vi "Esclatometre_USB.vi"() -> ()   [LabVIEW 2017]
doc: "Esclatometre_USB - Versió Esclatòmetre feta sobre una base de Conus USB"
uses:
  Control 1.ctl
  Program Files/National Instruments/LabVIEW 2017/ProjectTemplates/Source/Core/Simple State Machine/controls/Data.ctl
  Program Files/National Instruments/LabVIEW 2017/ProjectTemplates/Source/Core/Simple State Machine/controls/StateEsclatometre.ctl
  <vilib>/DAQmx/read.llb/DAQmx Read (Digital 1D Bool NChan 1Samp 1Line).vi
  <vilib>/DAQmx/write.llb/DAQmx Write (Digital 1D Bool NChan 1Samp 1Line).vi
  <vilib>/DAQmx/miscellaneous.llb/DAQmx Fill In Error Info.vi
  Instance           2 17Saved   Conus_USB .vi
  Instance           1 17Saved   Conus_USB .vi
  Instance           4 17Saved   Conus_USB .vi
  <vilib>/Utility/file.llb/Write Delimited Spreadsheet (DBL).vi
panel:
  out "TextTemps":string
  out "TextDefor":string caption="TextDeformacio"
  out "FactorsUnitatsTermesInp_D":dbl[](array[numeric]) caption="FactorsUnitatsPendents_D"
  out "FactorsUnitatsTermesInd":dbl[](array[numeric]) caption="FactorsUnitatsPendents_F"
  out "TermesInd":dbl[](array[numeric]) caption="Pendents" format="%#_8g"
  in  "BtMaxD":bool caption="BtMaxF"
  out "MaximDaFmax":sgl caption="Maxim"
  out "ArraiMaxF_D":dbl[][](array[numeric])
  out "ArraiMaxims":sgl[](array[numeric])
  in  "Activa cilindre":bool
  out "data 2":bool[](array[boolean])
  out "Calibrar":bool
  out "Paro Emergencia":bool caption="Emergencia"
  out "Valor de control Paro Rotura":dbl caption="Valor de control sobrecarga"
  out "data":bool[](array[boolean])
  out "Data":T1
  out "Cilindre":bool caption="Pujar"
  in  "Rep. Fetes":u8 caption="N. Rep."
  in  "Salir":bool
  in  "EtiquetaTipusParo":string caption="N. Rep."
  in  "Etiqueta Velocitats":string caption="Presión"
  out "appended array":refnum<vi>[](array[refnum])
  out "MissatgesUsuari":string[](array[string])
  out "Caselles":refnum<vi>[](array[refnum])
  out "StringsEstatMáquina":string[](array[string])
  out "ParoDefor":bool caption="ParoRotura"
  out "ParoDeforFet":bool caption="ParoProcessat"
  out "ParoCargaFet":bool caption="ParoProcessat"
  out "ParoCarga":bool caption="ParoProcessat"
  in  "CaptadorD":u16(ring) caption="Unidades" items=["Tiempo"]
  in  "ActivaParoRotura":T2
  in  "ValorParoRotura":sgl caption="Rotura (%)" min=0 format="%#_3f"
  out "Ensayo activo":bool caption="Prueba en curso"
  out "ArraiMostresxProva":dbl[](array[numeric])
  out "NMostres":dbl
  in  "BtEliminarUltima":bool=TRUE caption="Eliminar última"
  out "Estado ensayo:":string caption="Tiempo"
  out "CodiAturada":u32
  out "ViuMotor":bool
  out "MotorBipolar":bool
  out "Baixar":bool
  out "Pujar":bool
  out "PrimerCaptador":i32
  out "rings":refnum<vi>[](array[refnum])
  in  "IndexUnitatsD":u8
  in  "IndexUnitatsF":u8
  in  "IndexCaptadorD":u8
  in  "IndexCaptadorF":u8
  out "EtiquetesRegistre":string[](array[string])
  out "Active_motor":bool
  in  "IniciAssaig":bool caption="Inici x Boto"
  out "DeforActiu":bool caption="Extensòmetre Pot."
  out "ValorSenseTara":dbl
  in  "VelocitatMàxima":dbl
  in  "BtMaxF":bool
  in  "CaptadorF":u16(ring) caption="Unidades" items=["P-40 bar"=22, "No presente"=25]
  in  "UnidadesF":u16(ring) caption="Unidades" items=["bar"=7, "kg/cm2"=8]
  in  "BtTaraF":bool caption="TARA"
  out "Fuerza":sgl caption="Presión" format="%.2f"
  out "Nº Tests":u8 caption="Tests:"
  out "Sobrecarga":bool
  out "Paro Manual":bool
  out "FCI":bool caption="FCR"
  out "FCS":bool caption="FCA"
  in  "ResoExten":i8(ring) caption="Resolució Extensometre" items=["0.1", "0.2", "0.5", "0.01", "0.02", "0.05", "0.001", "0.002", "0.005"]
  out "PrecargaOn":bool
  in  "ValorPrecarga":dbl caption="Precarga (%)"
  out "Calibratge D":dbl[](array[numeric])
  in  "UnidadesD":u16(ring) caption="Unidades" items=["sg"]
  in  "BtTaraD":bool caption="TARA"
  out "Deformacion":sgl caption="Tiempo" format="%.1f"
  out "Celula_0":u8
  in  "Células":u8(ring) caption="Célula 1" items=["0.5 kg", "1 Kg", "2 Kg", "5 kg", "10 kg", "20 kg", "50 kg", "100 kg", "200 kg", "300 kg", "500 kg", "1000 kg", "2000 kg", "5000 kg", "10000 kg", "20000 kg", "30000 kg", "P-20 kg", "P-200 kg", "P-500 kg", "P-5000 kg", "P-20000 kg", "P-40 bar", "P-60 bar", "P-20 bar", "No presente"]
  in  "UnidadesF_C2":u16(ring) caption="Unidades" items=["bar"=7]
  in  "UnidadesF_C1":u16(ring) caption="Unidades" items=["bar"=7, "kg/cm2"=8]
  out "ArraiUnitats":cluster{"String":string, "Value":u16}[](array[cluster])=[{"String"="kg", "Value"=0}, {"String"="N", "Value"=1}, {"String"="g", "Value"=2}, {"String"="daN", "Value"=3}, {"String"="cN", "Value"=4}, {"String"="KN", "Value"=5}, {"String"="lb", "Value"=6}]
  in  "UnitatsF":u8[](array[numeric])
  in  "Velocidad Retorno":sgl caption="Retorno" min=1 max=240 step=1 format="%#.1f"
  in  "Velocidad Ensayo":sgl caption="Ensayo" min=0 max=240 step=1
  out "ValorSobrecargaC2":dbl
  out "Valor de control sobrecarga":dbl
  out "Calibratge":dbl[](array[numeric])
  in  "ParaAssaig":bool
  out "ParoProcessat":bool
  out "Salidas_mando":T3={"HI_down"=TRUE, " LO_down"=TRUE, "HI_up"=TRUE, "*"=TRUE, " LO_up"=TRUE, " start"=TRUE, " Ensayo_down"=TRUE, " Ensayo_up"=TRUE}
  out "TempsLectura":u32=150
  out "Maxim":sgl
  in  "Inhibicio":bool
  in  "Ensayonuevo":bool caption="Ensayo Nuevo"
  in  "Guardar":bool caption="Informe"
  out "Iniciar / Finalizar":bool=TRUE caption="Finalizar prueba"
  out "TablaFinal":dbl[][](array[numeric])
  out "Tabla":dbl[][](array[numeric])
  in  "Columna":i32
  out "Paro Emergencia":bool
  out "ParoRotura":bool
  out "AssaigMM":bool
  out "DSenseTara":sgl caption="Fuerza - N"
  out "FactorsUnitatsPendents_D":dbl[](array[numeric])
  out "ConversioUnitatsD":dbl[](array[numeric])=[1.0, 9.8756, 1000.0, 0.98]
  in  "DadesAdquirides":dbl[](array[numeric]) format="%#_8g"
  out "FactorsUnitatsPendents_F":dbl[](array[numeric])
  in  "LedAssaig":bool caption="Ensayo Preparado"
  out "BaixarMM":bool
  out "PujarMM":bool
  in  "TaraD":sgl
  in  "ValMax":bool
  out "FSenseTara":sgl caption="Fuerza - N"
  in  "TaraF":sgl
  out "Password":string
  out "ValorSobrecargaC1":dbl
  out "ConversioUnitatsF":dbl[](array[numeric])=[1.0, 9.8756, 2.2]
  out "Pendents":dbl[](array[numeric]) format="%#_8g"
  in  "Procesa datos":bool
  in  "Stop":bool=TRUE
  in  "First time":bool
  out "?":cluster{"Y":dbl[], "Y":dbl[]}[](graph)
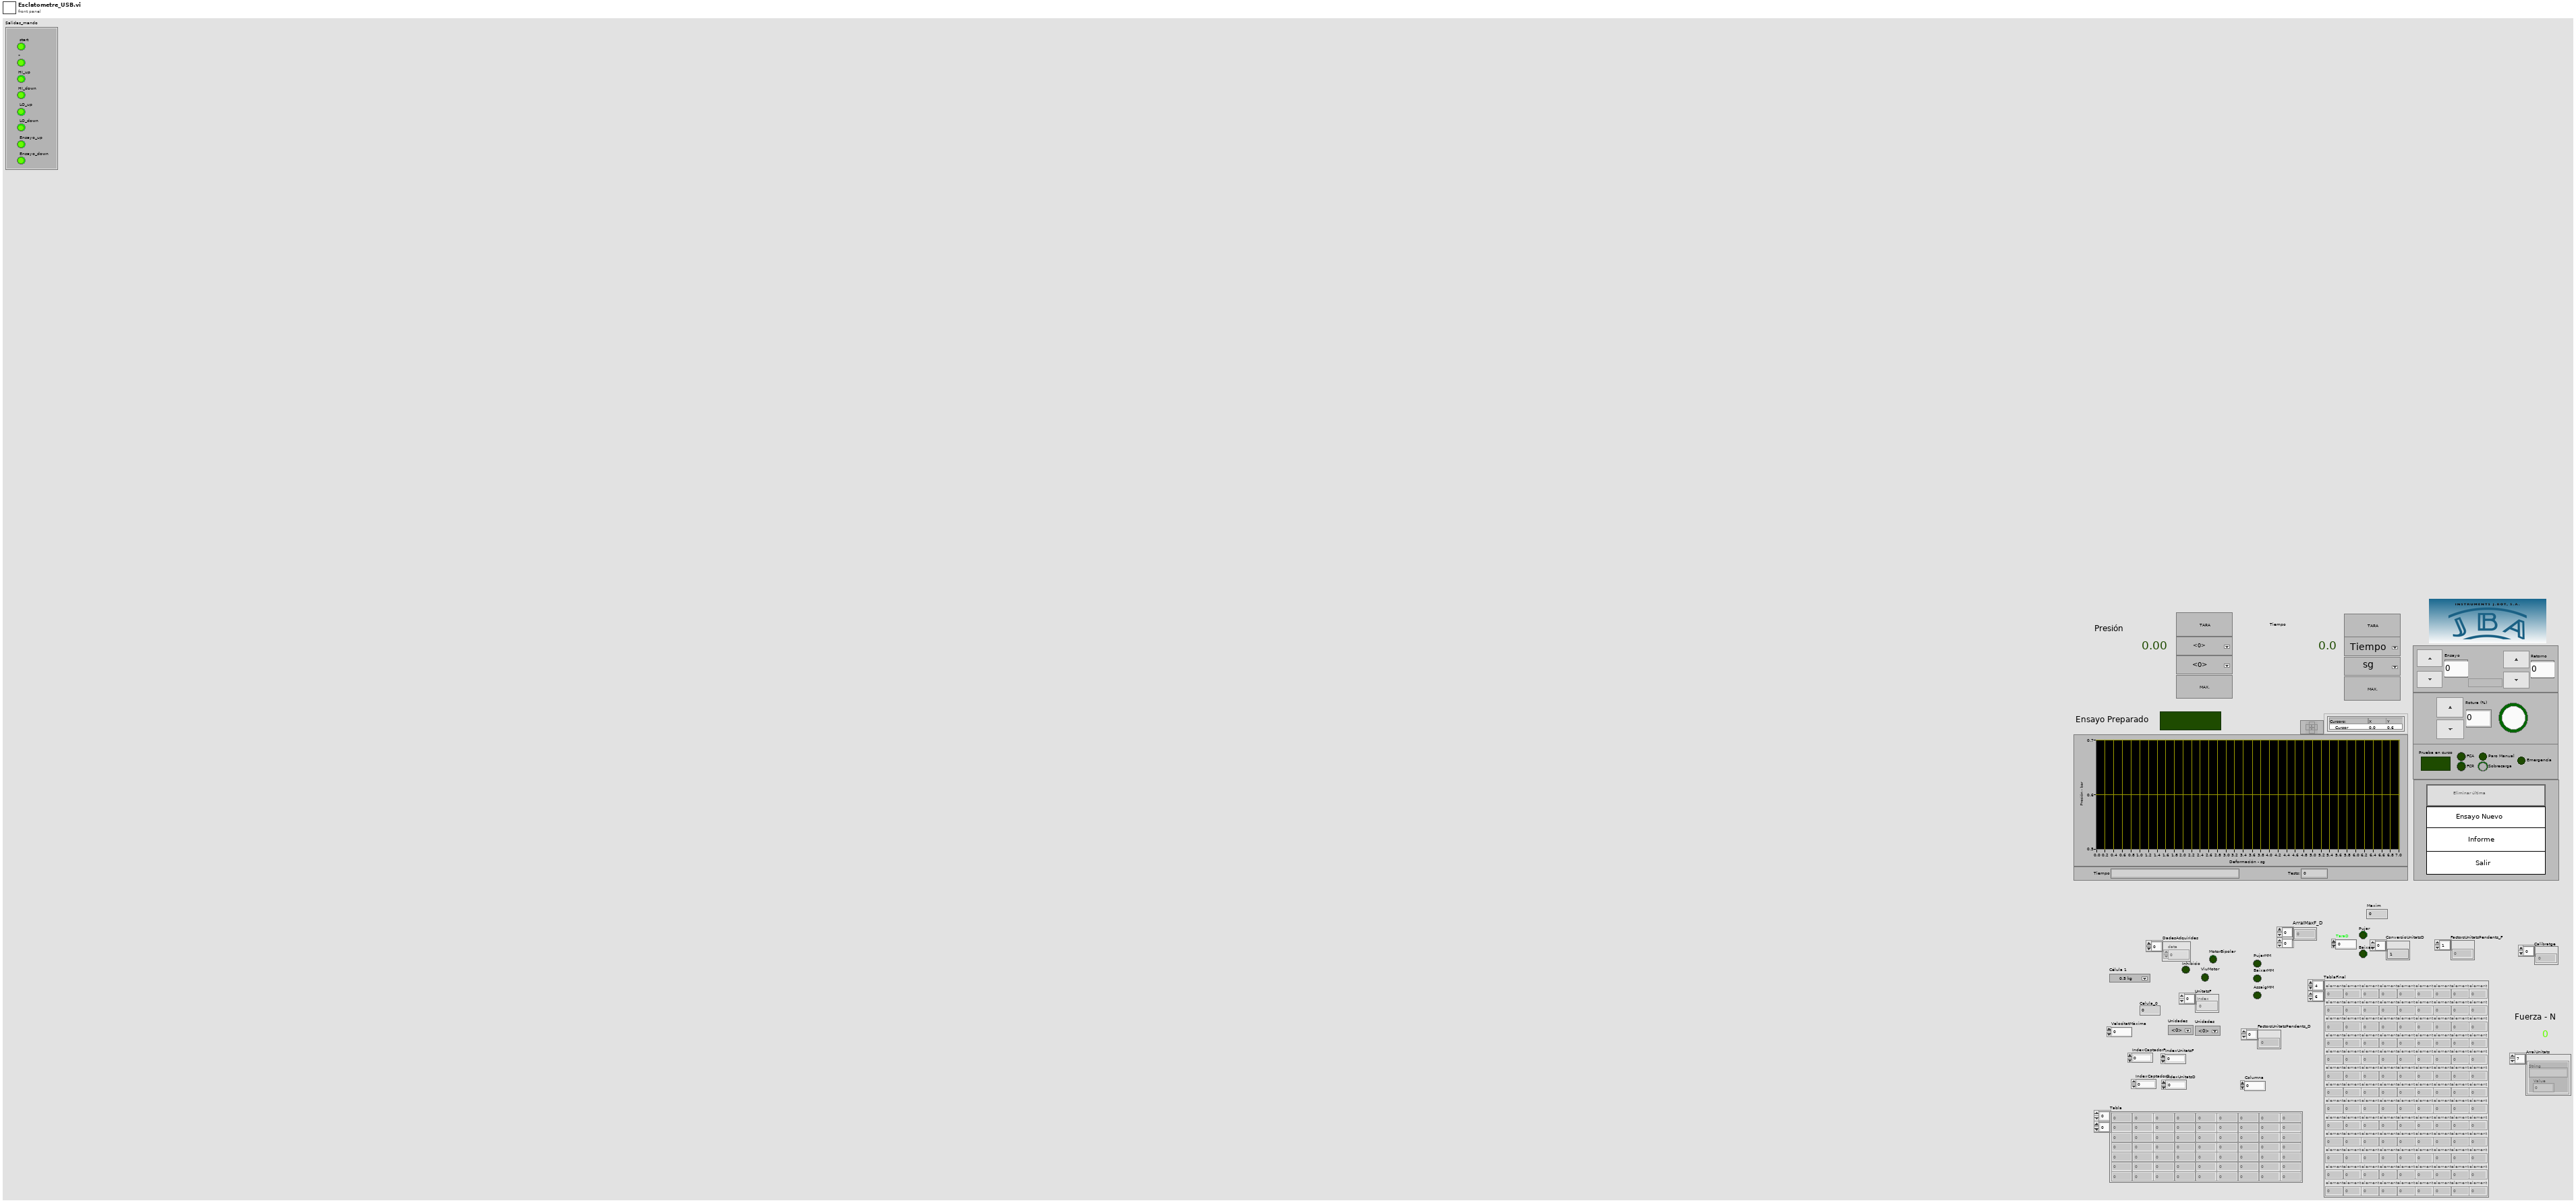
[diagram p1: front panel]
types:
  T1 = typedef "Data.ctl" = cluster{"Boolean <Replace Me>":bool, "String <Replace Me>":string, "Numeric <Replace Me>":dbl}
  T2 = typedef "Control 1.ctl" = bool
  T3 = cluster{"HI_down":bool, " LO_down":bool, "HI_up":bool, "*":bool, " LO_up":bool, " start":bool, " Ensayo_down":bool, " Ensayo_up":bool}
  T4 = typedef "StateEsclatometre.ctl" = enum16{"Initialize", "Wait for Event", "EsperaAssaig", "IniciaAssaig", "Assaig", "FiAssaig", "Emergencia", "Exit"}
  T5 = typedef "LVStringsAndValuesArrayTypeDef_U8.ctl" = cluster{"String":string, "Value":u8}[]
  T6 = typedef "LVStringsAndValuesArrayTypeDef_U16.ctl" = cluster{"String":string, "Value":u16}[]
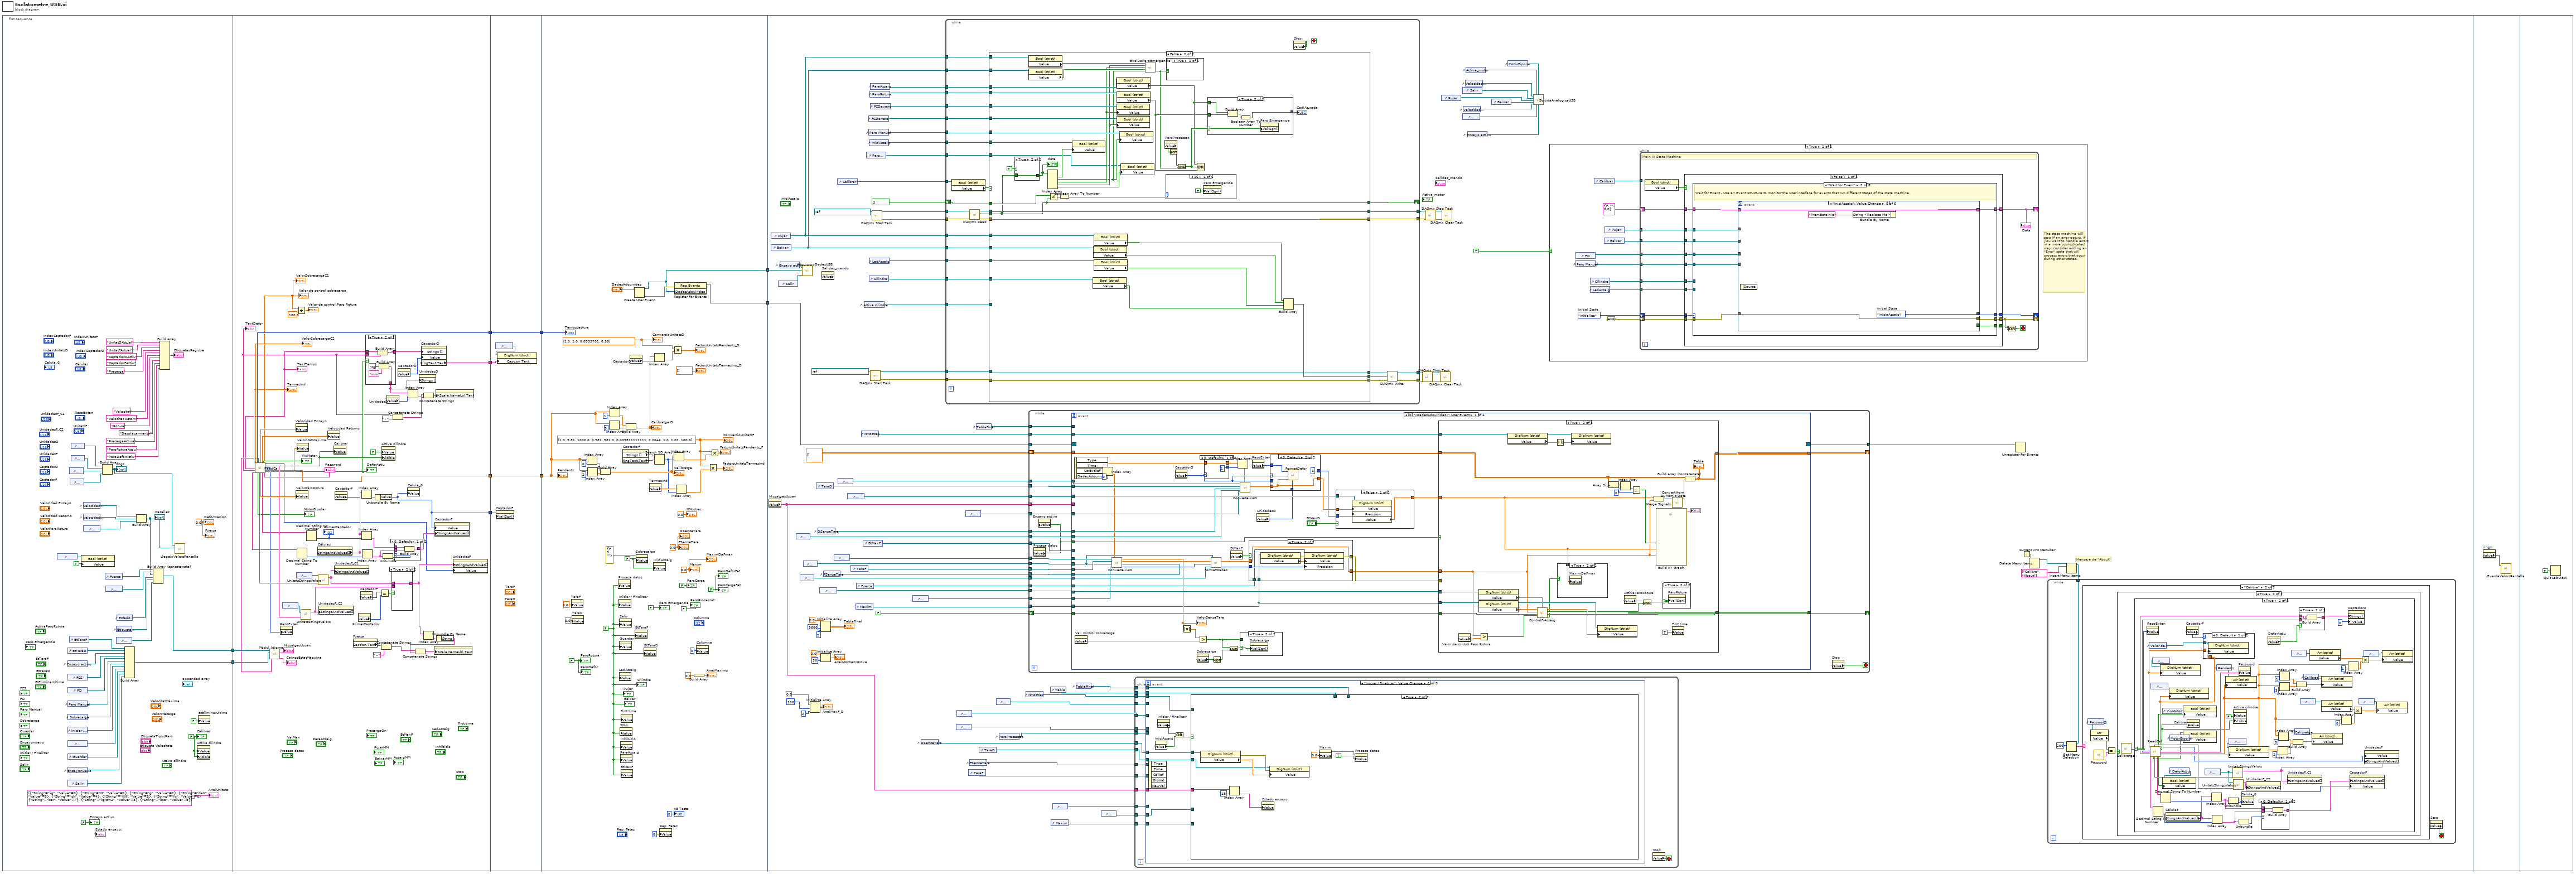
[diagram p0: block diagram]
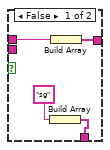
[diagram p3: hidden frame]
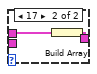
[diagram p4: hidden frame]
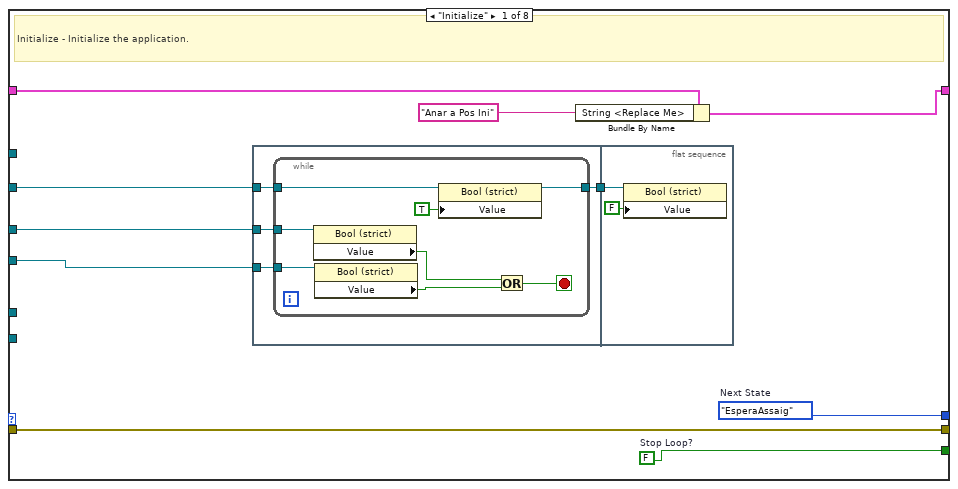
[diagram p6: hidden frame]
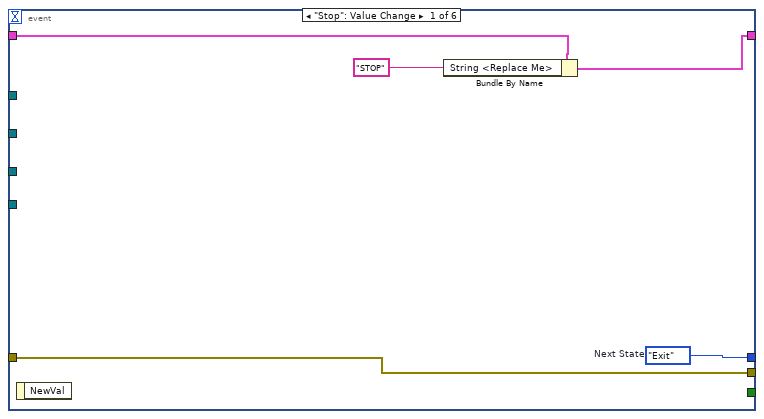
[diagram p7: hidden frame]
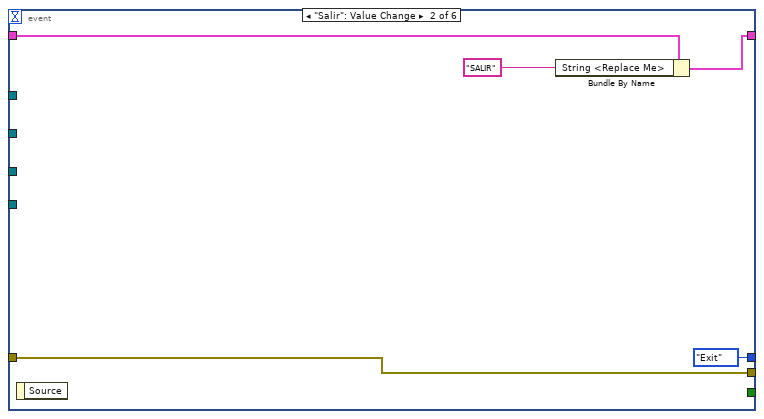
[diagram p8: hidden frame]
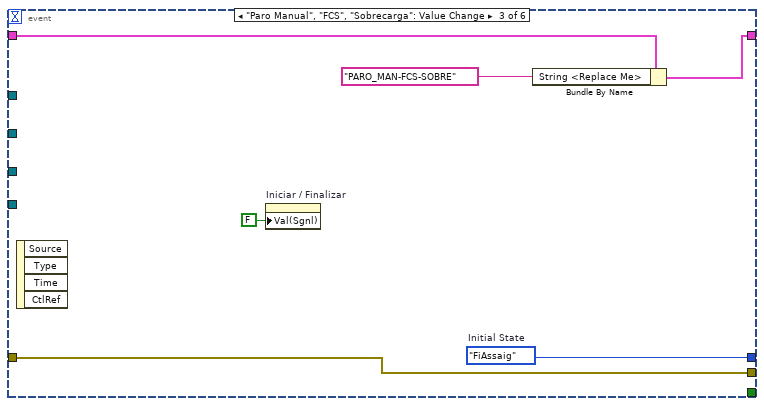
[diagram p9: hidden frame]
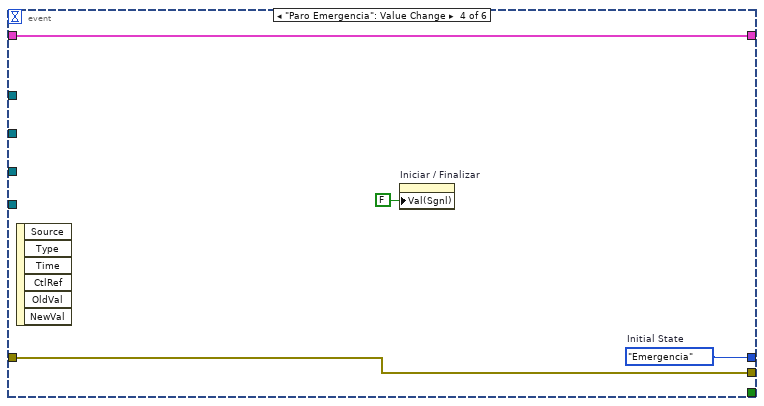
[diagram p10: hidden frame]
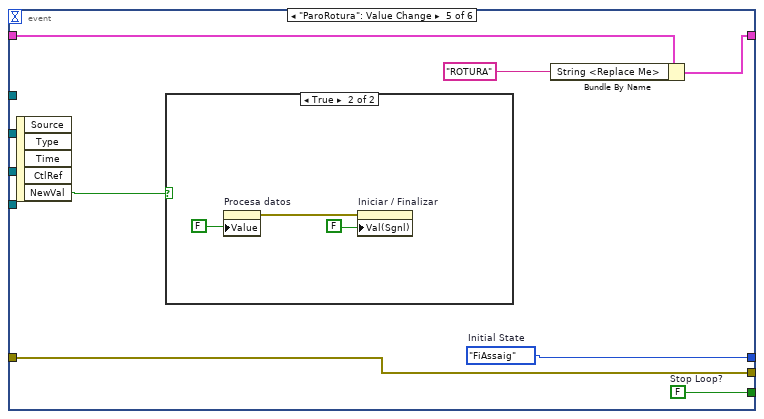
[diagram p11: hidden frame]
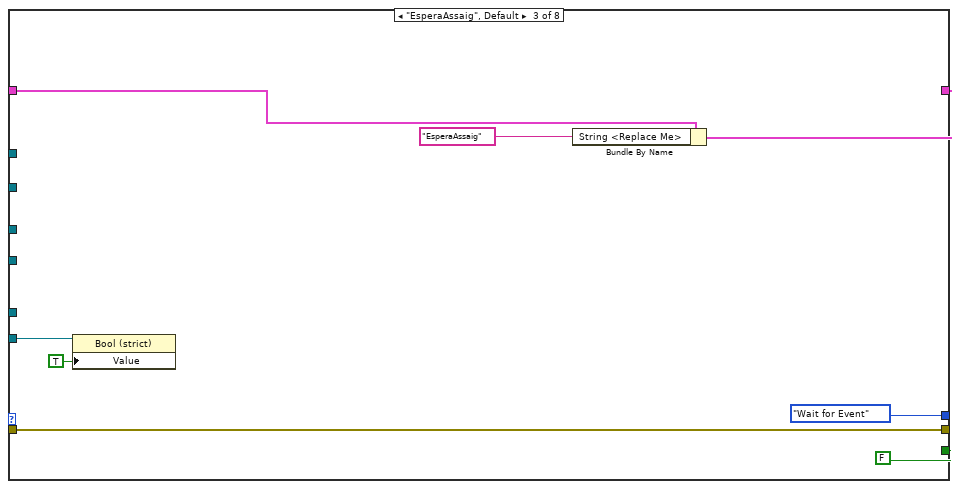
[diagram p13: hidden frame]
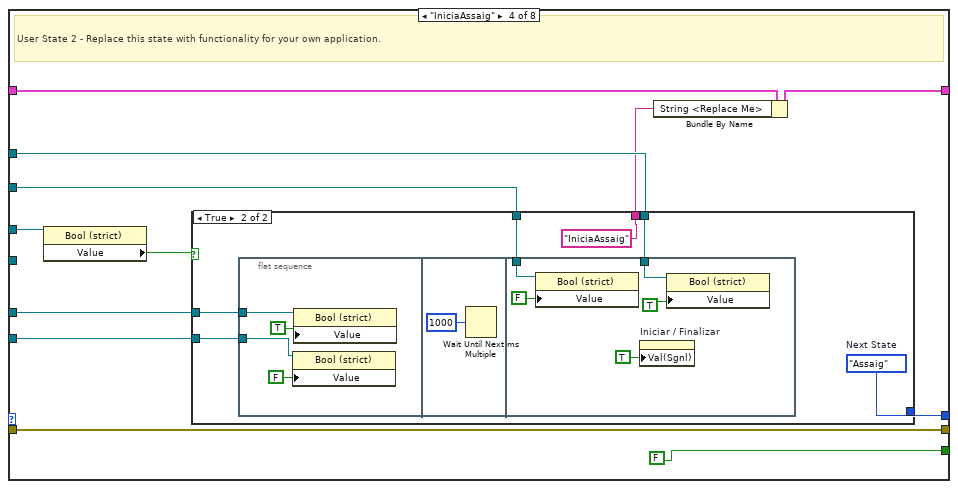
[diagram p14: hidden frame]
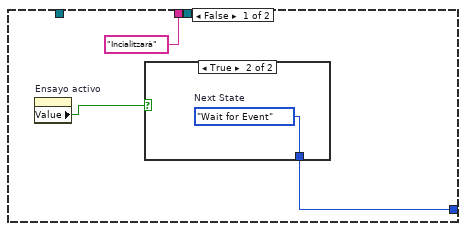
[diagram p15: hidden frame]
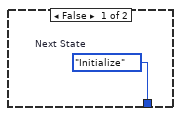
[diagram p16: hidden frame]
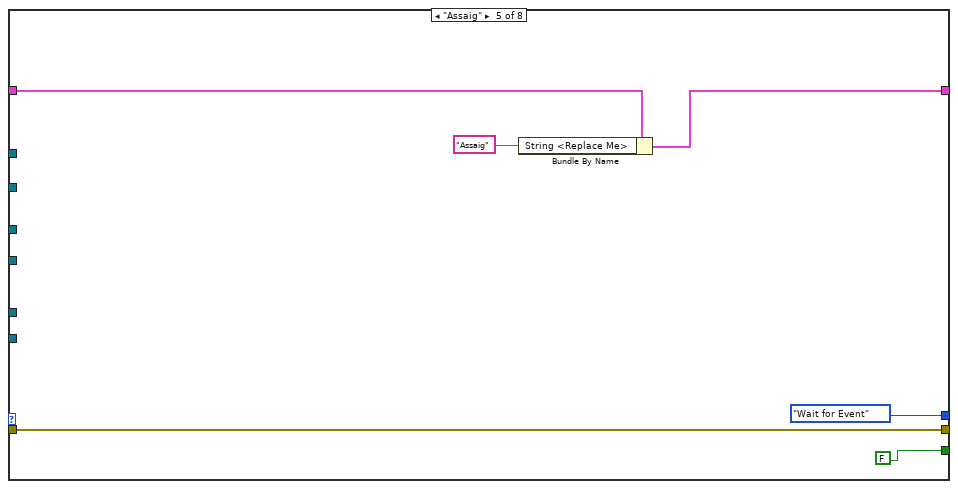
[diagram p17: hidden frame]
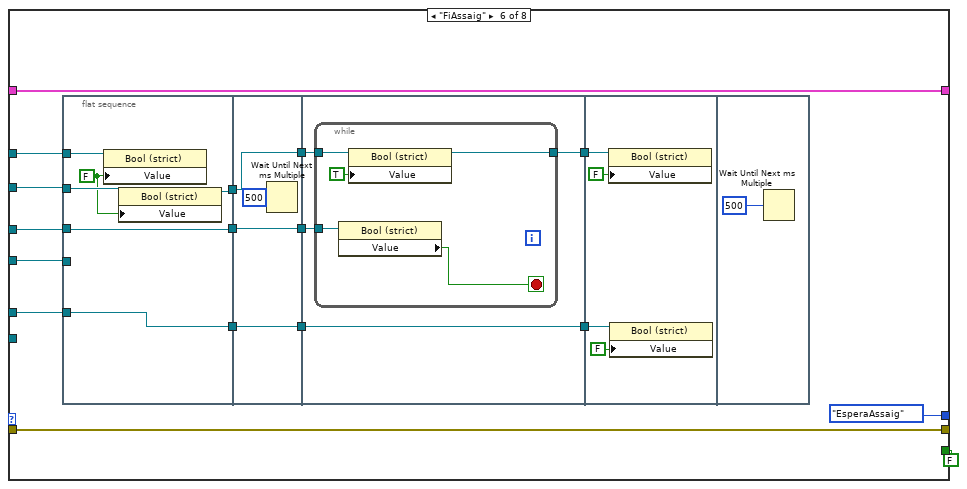
[diagram p18: hidden frame]
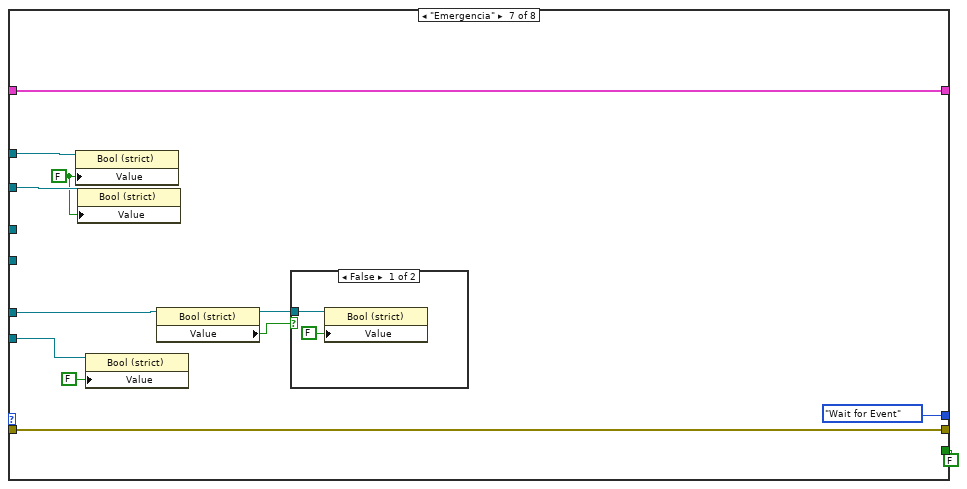
[diagram p19: hidden frame]
diagram:
  n1 = flat-sequence {
    tunnel: [w22] -> w3
    tunnel: [w21] -> w2
    tunnel: [w105] -> w10
    tunnel: [w118] -> w9
    tunnel: [w79] -> w4
    tunnel: w3 -> [w73]
    tunnel: w2 -> [w74]
    tunnel: [w58] -> w1
    tunnel: w10 -> [w142]
    tunnel: [w142] -> w8
    tunnel: w9 -> [w141]
    tunnel: [w141] -> w7
    tunnel: w4 -> [w140]
    tunnel: w1 -> [w138]
    tunnel: w8 -> [w167]
    tunnel: [w186] -> w6
    tunnel: [w178] -> w5
    tunnel: w7 -> [w177]
    tunnel: w6 -> [w276]
    tunnel: w5 -> [w258]
    frame #0 {
      w11 = FALSE ("Calibrar")
      w15 = sgl 0.0 ("Deformacion")
      (unwired) "CaptadorFActiu" ("value")
      n2 = control-ref of="ActivaParoRotura"() -> (w13:refnum<vi>)
      n3 = control-ref of="BtTaraD"() -> (w37:refnum<vi>)
      n4 = control-ref of="Ensayo activo"() -> (w36:refnum<vi>)
      n5 = control-ref of="FCS"() -> (w35:refnum<vi>)
      n6 = control-ref of="FCI"() -> (w34:refnum<vi>)
      n7 = control-ref of="Paro Manual"() -> (w33:refnum<vi>)
      n8 = control-ref of="Sobrecarga"() -> (w32:refnum<vi>)
      n9 = control-ref of="Iniciar / Finalizar"() -> (w31:refnum<vi>)
      n10 = control-ref of="BtEliminarUltima"() -> (w30:refnum<vi>)
      n11 = control-ref of="Guardar"() -> (w20:refnum<vi>)
      n12 = control-ref of="Ensayonuevo"() -> (w29:refnum<vi>)
      n13 = control-ref of="Salir"() -> (w28:refnum<vi>)
      n14 = control-ref of="BtTaraF"() -> (w38:refnum<vi>)
      n15 = control-ref of="CaptadorD"() -> (w42:refnum<vi>)
      n16 = control-ref of="CaptadorF"() -> (w41:refnum<vi>)
      n17 = control-ref of="UnidadesD"() -> (w44:refnum<vi>)
      n18 = control-ref of="UnidadesF"() -> (w43:refnum<vi>)
      n19 = property class="Bool (strict)"(reference=w13, "Value"=T2 TRUE) -> ()  [unwired: 1 in, 2 out]
      n20 = control-ref of="Velocidad Ensayo"() -> (w27:refnum<vi>)
      n21 = control-ref of="Velocidad Retorno"() -> (w45:refnum<vi>)
      n22 = control-ref of="ValorParoRotura"() -> (w26:refnum<vi>)
      n23 = Build Array(w44, w43, w42, w41) -> (w40:refnum<vi>[])
      "rings" <- w40
      n24 = control-ref of="Fuerza"() -> (w25:refnum<vi>)
      n25 = control-ref of="Deformacion"() -> (w24:refnum<vi>)
      n26 = control-ref of="Etiqueta Velocitats"() -> (w17:refnum<vi>)
      n27 = control-ref of="EtiquetaTipusParo"() -> (w16:refnum<vi>)
      n28 = control-ref of="Estado ensayo:"() -> (w18:refnum<vi>)
      n29 = Build Array(w38, w37, w36, w35, w34, w33, w32, w31, w30, w20, w29, w28) -> (w22:refnum<vi>[])
      n30 = Build Array(w27, w45, w26) -> (w19:refnum<vi>[])
      "Caselles" <- w19
      n31 = Build Array (concatenate)(w25, w24, w19, w18, w17, w16) -> (w21:refnum<vi>[])
      n32 = Build Array("UnitatDActual" ("value"), "UnitatFActual" ("value"), "CaptadorDActiu" ("value"), "Precarga" ("value"), "Velocitat" ("value"), "Velocitat Retorn" ("value"), "Rotura" ("value"), "Desplazamiento" ("value"), "PrecargaActiva" ("value"), "ParoRoturaActiu" ("value"), "ParoDeforActiu" ("value")) -> (→"EtiquetesRegistre":string[])
      n33 = call "LlegeixValorsPantalla.vi"("rings"=w40, "Caselles 2"=w19) -> ()  [unwired: 9 in]
      n34 = property on="Activa cilindre" class="Bool (strict)"("Value"=w11, "Visible"=w11) -> ()  [unwired: 2 in, 2 out]
      n35 = property on="BtEliminarUltima" class="Bool (strict)"("Value"=FALSE ("BtEliminarUltima")) -> ()  [unwired: 2 in, 2 out]
      "Ensayo activo" <- FALSE ("Ensayo activo")
      "Fuerza" <- w15
      "Deformacion" <- w15
      "ArraiUnitats" <- cluster{"String":string, "Value":u16}[] [{"String"="kg", "Value"=0}, {"String"="N", "Value"=1}, {"String"="g", "Value"=2}, {"String"="daN", "Value"=3}, {"String"="cN", "Value"=4}, {"String"="KN", "Value"=5}, {"String"="lb", "Value"=6}, {"String"="bar", "Value"=7}, {"String"="kg/cm2", "Value"=8}, {"String"="kpa", "Value"=9}] ("Strings And Values [] 2")
      "Calibrar" <- w11
    }
    frame #1 {
      n36 = call "ReadCal.vi"() -> ("SobrecargaC2"=→"ValorSobrecargaC2":dbl, "TermesInd"=→"TermesInd":dbl[], "ResoExten"=w104:i8, "TextTemps"=w60:string, "TextDefor"=w59:string, "SegonCaptador"=w111:string, "TempsLectura"=w118:u16, "Idioma"=w62:string, "MotorBipolar"=→"MotorBipolar":bool, "UnitatsC2"=w112:string, "UnitatsC1"=w113:string, "Velocitat"=w119:dbl, "ParoRotura"=w120:dbl, "V. Retorn"=w70:dbl, "PrimerCaptador"=w109:string, "ViuMotor"=→"ViuMotor":bool, "DeforActiva"=w63:bool, "Unidades"=w71:u8, "Calibrar"=w66:bool, "SobrecargaC1"=w69:dbl, "Password"=→"Password":string, "Pendents"=w105:dbl[], "VelocitatMàxima"=w102:dbl)  [unwired: 2 in, 3 out]
      "ValorSobrecargaC1" <- w69
      "Valor de control sobrecarga" <- w69
      "DeforActiu" <- w63
      "TextDefor" <- w59
      "TextTemps" <- w60
      n37 = call "Módul_Idioma.vi"("Idioma"=w62, "Array"=w73, "Caselles"=w74) -> ("TextosEstatMaquina"=→"StringsEstatMáquina":string[], "MissatgesUsuari"=→"MissatgesUsuari":string[])  [unwired: 7 in]
      n38 = property on="ResoExten" class="Ring (strict)"("Value"=w104) -> ()  [unwired: 2 in, 2 out]
      n39 = control-ref of="ArraiUnitats"() -> (w114:refnum<vi>)
      n40 = property on="Velocidad Ensayo" class="DigNum (strict)"("Value"=w119) -> ()  [unwired: 2 in, 2 out]
      n41 = property on="ValorParoRotura" class="DigNum (strict)"("Value"=w120) -> ()  [unwired: 2 in, 2 out]
      n42 = Divide(x=w69, y=100.0) -> (x/y=→"Valor de control Paro Rotura":dbl)
      n43 = control-ref of="ArraiUnitats"() -> (w115:refnum<vi>)
      n44 = property on="VelocitatMàxima" class="DigNum (strict)"("Value"=w102) -> ()  [unwired: 2 in, 2 out]
      n45 = Decimal String To Number(string=w111) -> (number=w110:i32)  [unwired: 2 in, 1 out]
      n46 = call "UnitatsStringsValors.vi"("UnitatsC1"=w112, "Arr Refnum"=w114) -> ("Array 2"=w88:cluster{"String":string, "Value":u16}[])  [unwired: 1 out]
      n47 = Decimal String To Number(string=w109) -> (number=w108:i32)  [unwired: 2 in, 1 out]
      "PrimerCaptador" <- w108
      n48 = property on="Células" class="Ring (strict)"() -> ("StringsAndValues[]"=w95:T5)  [unwired: 2 in, 2 out]
      n49 = call "UnitatsStringsValors.vi"("UnitatsC1"=w113, "Arr Refnum"=w115) -> ("Array 2"=w89:cluster{"String":string, "Value":u16}[])  [unwired: 1 out]
      n50 = property on="UnidadesF_C2" class="Ring (strict)"("StringsAndValues[]"=w88) -> ()  [unwired: 2 in, 2 out]
      n51 = property on="Velocidad Retorno" class="DigNum (strict)"("Value"=w70) -> ()  [unwired: 2 in, 2 out]
      n52 = property on="Calibrar" class="Bool (strict)"("Value"=w66) -> ()  [unwired: 2 in, 2 out]
      n53 = property on="UnidadesF_C1" class="Ring (strict)"("StringsAndValues[]"=w89) -> ()  [unwired: 2 in, 2 out]
      n54 = property on="CaptadorF" class="Ring (strict)"() -> ("Value"=w93:u16)  [unwired: 2 in, 2 out]
      n55 = property on="Fuerza" class="DigNum (strict)"() -> ("Caption.Text"=w100:string)  [unwired: 2 in, 2 out]
      n56 = property on="PrimerCaptador" class="DigNum (strict)"() -> ("Value"=w90:i32)  [unwired: 2 in, 2 out]
      n57 = property on="CaptadorF" class="Ring (strict)"() -> ("Value"=w91:u16)  [unwired: 2 in, 2 out]
      n58 = Index Array(array=w95, index=w93) -> (element=w94:cluster{"String":string, "Value":u8})
      n59 = Index Array(array=w95, index=w108) -> (element=w97:cluster{"String":string, "Value":u8})
      n60 = Index Array(array=w95, index=w110) -> (element=w106:cluster{"String":string, "Value":u8})
      n61 = case shown="True" w63 {
        tunnel: w60 -> [w123 w128]
        tunnel: [w126 w132] -> w84
        tunnel: w59 -> [_ w127]
        tunnel: [w124 w129] -> w61
        frame False {
          n62 = Build Array("sg") -> (w124:string[])
          n63 = Build Array(w123) -> (w126:string[])
        }
        frame True {
          n64 = Build Array(w128, w127) -> (w132:string[])
          n65 = Build Array("sg", "mm") -> (w129:string[])
        }
      }
      n66 = Unbundle By Name(w94) -> ("Value"=w79:u8)
      n67 = Equal?(x=w91, y=w90) -> (x = y?=w92:bool)
      n68 = Concatenate Strings(w100, " - ") -> (w99:string)
      n69 = property on="Activa cilindre" class="Bool (strict)"("Value"=FALSE ("ActivaCilindre"), "Visible"=w66) -> ()  [unwired: 2 in, 2 out]
      n70 = Unbundle(w106) -> ("Value"=w107:u8)  [unwired: 1 out]
      n71 = property on="UnidadesD" class="Ring (strict)"() -> ("Value"=w83:u16)  [unwired: 2 in, 2 out]
      n72 = case shown="True" w92 {
        tunnel: w89 -> [_ w122]
        tunnel: [w121 w122] -> w72
        tunnel: w88 -> [w121 _]
        frame False {
        }
        frame True {
        }
      }
      n73 = Concatenate Strings(w59, " - ") -> (w80:string)
      n74 = case shown="0, Default" w107 {
        tunnel: w97 -> [w135 w136]
        tunnel: w106 -> [w134 _]
        tunnel: [w133 w137] -> w96
        frame 0, Default {
          n75 = Build Array(w135, w134) -> (w133:cluster{"String":string, "Value":u8}[])
        }
        frame 17 {
          n76 = Build Array(w136) -> (w137:cluster{"String":string, "Value":u8}[])
        }
      }
      n77 = property on="CaptadorD" class="Ring (strict)"() -> ("Value"=w85:u16)  [unwired: 2 in, 2 out]
      n78 = property on="Celula_0" class="DigNum (strict)"("Value"=w79) -> ()  [unwired: 2 in, 2 out]
      n79 = Index Array(array=w61, index=w83) -> (element=w82:string)
      n80 = property on="UnidadesD" class="Ring (strict)"("Strings []"=w61) -> ()  [unwired: 2 in, 2 out]
      n81 = property on="CaptadorD" class="Ring (strict)"("Strings []"=w84, "Value"=w85) -> ("RingText.Text"=w58:string)  [unwired: 2 in, 2 out]
      n82 = Concatenate Strings(w80, w82) -> (w98:string)
      n83 = Index Array(array=w72) -> (element=w86:cluster{"String":string, "Value":u16})  [unwired: 1 in]
      n84 = property on="CaptadorF" class="Ring (strict)"("Value"=w79, "StringsAndValues[]"=w96) -> ()  [unwired: 2 in, 2 out]
      n85 = property class="XYGraph (strict)"("XScale.NameLbl.Text"=w98) -> ()  [unwired: 2 in, 2 out]
      n86 = Unbundle By Name(w86) -> ("String"=w87:string)
      n87 = Concatenate Strings(w99, w87) -> (w103:string)
      n88 = property class="XYGraph (strict)"("YScale.NameLbl.Text"=w103) -> ()  [unwired: 2 in, 2 out]
      n89 = property on="UnidadesF" class="Ring (strict)"("StringsAndValues[]"=w72, "Value"=w71) -> ()  [unwired: 2 in, 2 out]
    }
    frame #2 {
      n90 = control-ref of="Deformacion"() -> (w139:refnum<vi>)
      n91 = property on="CaptadorF" class="Ring (strict)"("Val(Sgnl)"=w140) -> ()  [unwired: 2 in, 2 out]
      n92 = property class="DigNum (strict)"(reference=w139, "Caption.Text"=w138) -> ()  [unwired: 1 in, 2 out]
    }
    frame #3 {
      w155 = FALSE ("ParoCargaFet")
      w149 = sgl 0.0 ("Maxim")
      w154 = FALSE ("ParoRotura")
      w165 = dbl[] [1.0, 1.0, 0.0393701, 0.98]
      w180 = sgl 0.0 ("FSenseTara")
      w148 = dbl[] [1.0, 9.81, 1000.0, 0.981, 981.0, 0.009811111111, 2.2046, 1.0, 1.02, 100.0]
      w160 = FALSE ("Sobrecarga")
      w152 = FALSE ("Iniciar / Finalizar")
      n93 = property on="TaraF" class="DigNum (strict)"("Value"=sgl 0.0 ("Tara")) -> ()  [unwired: 2 in, 2 out]
      n94 = property on="TaraD" class="DigNum (strict)"("Value"=sgl 0.0 ("TaraD")) -> ()  [unwired: 2 in, 2 out]
      n95 = Index Array(array=w167, index=0) -> (element=w173:dbl)
      n96 = Index Array(array=w167, index=2) -> (element=w174:dbl)
      n97 = Build Array(w173, w174) -> (w172:dbl[])
      "Calibratge" <- w172
      n98 = Index Array(array=w167, index=3) -> (element=w168:dbl)
      n99 = Index Array(array=w167, index=1) -> (element=w166:dbl)
      n100 = property on="Procesa datos" class="Bool (strict)"("Value"=w152) -> ()  [unwired: 2 in, 2 out]
      n101 = property on="Iniciar / Finalizar" class="Bool (strict)"("Value"=w152) -> ()  [unwired: 2 in, 2 out]
      n102 = property on="LedAssaig" class="Bool (strict)"("Value"=w152) -> ()  [unwired: 2 in, 2 out]
      n103 = property on="Salir" class="Bool (strict)"("Value"=w152) -> ()  [unwired: 2 in, 2 out]
      n104 = property on="Guardar" class="Bool (strict)"("Value"=w152) -> ()  [unwired: 2 in, 2 out]
      n105 = property on="Stop" class="Bool (strict)"("Value"=w152) -> ()  [unwired: 2 in, 2 out]
      n106 = property on="Inhibicio" class="Bool (strict)"("Value"=w152) -> ()  [unwired: 2 in, 2 out]
      n107 = property on="ParaAssaig" class="Bool (strict)"("Value"=w152) -> ()  [unwired: 2 in, 2 out]
      n108 = property on="First time" class="Bool (strict)"("Value"=w152) -> ()  [unwired: 2 in, 2 out]
      n109 = property on="BtMaxF" class="Bool (strict)"("Value"=w152) -> ()  [unwired: 2 in, 2 out]
      n110 = property on="CaptadorF" class="Ring (strict)"() -> ("Strings []"=w159:string[], "RingText.Text"=w158:string)  [unwired: 2 in, 2 out]
      n111 = Build Array(w166, w168) -> (w163:dbl[])
      "Calibratge D" <- w163
      n112 = property on="CaptadorD" class="Ring (strict)"() -> ("Value"=w164:u16)  [unwired: 2 in, 2 out]
      n113 = Create User Event(user event datatype="DadesAdquirides") -> (user event=w178:refnum<user-event>, error out=w185:errorcluster)  [unwired: 1 in]
      n114 = property on="BtTaraF" class="Bool (strict)"("Value"=w152) -> ()  [unwired: 2 in, 2 out]
      n115 = property on="Sobrecarga" class="Bool (strict)"(error in=errorcluster {"status"=FALSE, "code"=0, "source"=""} ("error in (no error)"), "Value"=w160) -> ()  [unwired: 1 in, 2 out]
      n116 = property on="BtTaraD" class="Bool (strict)"("Value"=w152) -> ()  [unwired: 2 in, 2 out]
      n117 = property on="TermesInd" class="Arr (strict)"() -> ("Value"=w146:dbl[])  [unwired: 2 in, 2 out]
      n118 = property on="IniciAssaig" class="Bool (strict)"("Value"=w160) -> ()  [unwired: 2 in, 2 out]
      n119 = Index Array(array=w163, index=w164) -> (element=w162:dbl)
      n120 = Search 1D Array(1D array=w159, element=w158) -> (index of element=w145:i32)  [unwired: 1 in]
      n121 = property on="Rep. Fetes" class="DigNum (strict)"("Value"=u8 0 ("Rep. Fetes")) -> ()  [unwired: 2 in, 2 out]
      n122 = Multiply(x=w165, y=w162) -> (x*y=→"FactorsUnitatsPendents_D":dbl[])
      n123 = Index Array(array=w172, index=w145) -> (element=w171:dbl)
      n124 = register-events(error in=w185, w178) -> (reference out=w186:refnum<event-registration>)  [unwired: 1 in, 1 out]
      n125 = Index Array(array=w146, index=w145) -> (element=w144:dbl)
      n126 = Build Array(0.0 ("element")) -> (→"ArraiMaxims":dbl[])
      n127 = property on="Columna" class="DigNum (strict)"("Value"=0 ("Columna")) -> ()  [unwired: 2 in, 2 out]
      n128 = Multiply(x=w148, y=w144) -> (x*y=→"FactorsUnitatsTermesInd":dbl[])
      n129 = Multiply(x=w148, y=w171) -> (x*y=→"FactorsUnitatsPendents_F":dbl[])
      "Pendents" <- w167
      "ConversioUnitatsF" <- w148
      "FSenseTara" <- w180
      "ConversioUnitatsD" <- w165
      "DSenseTara" <- w180
      "ParoRotura" <- w154
      "Paro Emergencia" <- FALSE ("Paro Emergencia")
      "Maxim" <- w149
      "TempsLectura" <- w177
      "ParoProcessat" <- FALSE ("ParoProcessat")
      "Nº Tests" <- u8 0 ("Nº Tests")
      "Pujar" <- w152
      "Baixar" <- w152
      "NMostres" <- 0.0 ("NMostres")
      "ParoCarga" <- FALSE ("ValorCargaFet")
      "ParoCargaFet" <- w155
      "ParoDeforFet" <- w155
      "ParoDefor" <- w154
      "Cilindre" <- w152
      "MaximDaFmax" <- w149
      "FactorsUnitatsTermesInp_D" <- dbl[] [] ("FactorsUnitatsTermesInp_D")
    }
    frame #4 {
      # "Mensaje de \"About\""
      n130 = property on="MissatgesUsuari" class="Arr (strict)"() -> ("Value"=w214:string[])  [unwired: 2 in, 2 out]
      n131 = control-ref of="Pujar"() -> (w222:refnum<vi>)
      n132 = control-ref of="Baixar"() -> (w221:refnum<vi>)
      n133 = control-ref of="Salir"() -> (w259:refnum<vi>)
      n134 = control-ref of="Ensayo activo"() -> (w209:refnum<vi>)
      n135 = control-ref of="UnidadesD"() -> (w269:refnum<vi>)
      n136 = control-ref of="CaptadorF"() -> (w235:refnum<vi>)
      n137 = call "AdquisicioDadesUSB.vi"("Stop"=w259, "user event"=w258, "AssaigActiu"=w209) -> ()  [unwired: 9 in]
      n138 = control-ref of="UnidadesF"() -> (w268:refnum<vi>)
      n139 = Initialize Array(0.0 ("element"), 100 ("dimension size"), 2 ("dimension size")) -> (→"ArraiMaxF_D":dbl[][])
      n140 = control-ref of="TaraD"() -> (w272:refnum<vi>)
      n141 = control-ref of="DSenseTara"() -> (w273:refnum<vi>)
      n142 = control-ref of="ValorParoRotura"() -> (w265:refnum<vi>)
      n143 = Initialize Array(0.0 ("element"), 3600 ("dimension size"), 2 ("dimension size")) -> (→"TablaFinal":dbl[][])
      n144 = Initialize Array(0.0 ("element"), 30 ("dimension size")) -> (→"ArraiMostresxProva":dbl[])
      n145 = property on="Salidas_mando" class="Clust (strict)" props=["Value"]() -> ()  [unwired: 2 in, 3 out]
      n146 = control-ref of="FSenseTara"() -> (w278:refnum<vi>)
      n147 = control-ref of="FactorsUnitatsPendents_F"() -> (w277:refnum<vi>)
      n148 = control-ref of="Calibrar"() -> (w202:refnum<vi>)
      n149 = control-ref of="FactorsUnitatsPendents_D"() -> (w275:refnum<vi>)
      n150 = control-ref of="Deformacion"() -> (w274:refnum<vi>)
      n151 = control-ref of="TaraF"() -> (w279:refnum<vi>)
      n152 = control-ref of="Maxim"() -> (w257:refnum<vi>)
      n153 = control-ref of="Fuerza"() -> (w229:refnum<vi>)
      n154 = control-ref of="NMostres"() -> (w217:refnum<vi>)
      n155 = control-ref of="BtMaxF"() -> (w233:refnum<vi>)
      n156 = control-ref of="Activa cilindre"() -> (w201:refnum<vi>)
      n157 = control-ref of="Paro Emergencia"() -> (w203:refnum<vi>)
      n158 = control-ref of="FCDarrera"() -> (w240:refnum<vi>)
      n159 = control-ref of="Paro Manual"() -> (w239:refnum<vi>)
      n160 = control-ref of="IniciAssaig"() -> (w205:refnum<vi>)
      n161 = control-ref of="Cilindre"() -> (w208:refnum<vi>)
      n162 = control-ref of="LedAssaig"() -> (w207:refnum<vi>)
      n163 = control-ref of="ParoRotura"() -> (w238:refnum<vi>)
      n164 = control-ref of="ParaAssaig"() -> (w237:refnum<vi>)
      n165 = call <vilib>:"DAQmx Start Task.vi"("task/channels in"=refnum<k21> "Esclatometre_USBDigitalOut") -> ("task out"=w247:refnum<k21>, "error out"=w246:errorcluster)  [unwired: 13 in]
      n166 = control-ref of="FCDavant"() -> (w241:refnum<vi>)
      n167 = call <vilib>:"DAQmx Start Task.vi"("task/channels in"=refnum<k21> "Esclatometre_USBSDigitalIn") -> ("task out"=w254:refnum<k21>, "error out"=w253:errorcluster)  [unwired: 13 in]
      n168 = control-ref of="FactorsUnitatsTermesInd"() -> (w193:refnum<vi>)
      n169 = control-ref of="DSenseTara"() -> (w270:refnum<vi>)
      n170 = while {
        tunnel: w254 -> [w521]
        tunnel: w253 -> [w520]
        tunnel: [w540] -> w250
        tunnel: [w539] -> w249
        tunnel: w247 -> [w516]
        tunnel: w246 -> [w515]
        tunnel: [w512] -> w243
        tunnel: [w513] -> w242
        tunnel: w241 -> [w538]
        tunnel: w240 -> [w537]
        tunnel: w239 -> [w527]
        tunnel: w238 -> [w536]
        tunnel: w237 -> [w535]
        tunnel: w222 -> [w533]
        tunnel: w221 -> [w532]
        tunnel: w221 -> [w531]
        tunnel: w222 -> [w530]
        tunnel: w208 -> [w529]
        tunnel: w207 -> [w528]
        tunnel: w205 -> [w526]
        shift-right: [w525] -> _
        shift-left: bool[] [] ("data") -> [w509]
        tunnel: w203 -> [w524]
        tunnel: w202 -> [w523]
        tunnel: w201 -> [w508]
        stop <- w534 stop-if-true
        n171 = property class="Bool (strict)"(reference=w523) -> ("Value"=w522:bool)  [unwired: 1 in, 2 out]
        n172 = call-poly <vilib>:"DAQmx Read.vi"("task/channels in"=w521, "error in"=w520) -> ("task out"=w519:refnum<k21>, "data"=w517:bool[], "error out"=w518:errorcluster)  [unwired: 11 in]
        n173 = case shown="False" w522 {
          tunnel: w519 -> [w554 w572]
          tunnel: w518 -> [w553 w571]
          tunnel: [w554 w572] -> w540
          tunnel: [w553 w571] -> w539
          tunnel: w516 -> [w551 w569]
          tunnel: w515 -> [w550 w568]
          tunnel: [w550 w568] -> w511
          tunnel: [w551 w569] -> w514
          tunnel: w538 -> [w542 w601]
          tunnel: w537 -> [w546 w600]
          tunnel: w527 -> [_ w599]
          tunnel: w536 -> [_ w598]
          tunnel: w535 -> [_ w595]
          tunnel: w533 -> [_ w593]
          tunnel: w532 -> [_ w592]
          tunnel: w531 -> [_ w588]
          tunnel: w530 -> [_ w587]
          tunnel: w526 -> [_ w584]
          tunnel: w529 -> [_ w583]
          tunnel: w528 -> [_ w582]
          tunnel: [w547 w562] -> w525
          tunnel: w524 -> [w545 w574]
          tunnel: w517 -> [w547 w562]
          tunnel: [w552 w570] -> w510
          tunnel: w509 -> [_ w567]
          tunnel: w508 -> [w549 _]
          frame True {
            n174 = Index Array(array=w547) -> (element #3=w541:bool, element #4=w543:bool, element #5=w544:bool)  [unwired: 5 in, 2 out]
            n175 = property class="Bool (strict)"(reference=w546, "Value"=w543) -> ()  [unwired: 1 in, 2 out]
            n176 = property class="Bool (strict)"(reference=w545, "Value"=w544) -> ()  [unwired: 1 in, 2 out]
            n177 = property class="Bool (strict)"(reference=w542, "Value"=w541) -> ()  [unwired: 1 in, 2 out]
            n178 = property class="Bool (strict)"(reference=w549) -> ("Value"=w548:bool)  [unwired: 1 in, 2 out]
            n179 = Index Array(array=w547, index #1=0 ("index"), index #2=1 ("index")) -> (element #1=w559:bool, element #2=w558:bool)
            n180 = Build Array(w559, w558, FALSE ("element"), w548) -> (w552:bool[])
            "data 2" <- w547
          }
          frame False {
            n181 = case shown="True" TRUE {
              tunnel: w562 -> [_ w603]
              tunnel: [bool[] [FALSE, FALSE, FALSE, TRUE] ("data") w603] -> w561
              frame False {
              }
              frame True {
              }
            }
            "data" <- w561
            n182 = property class="Bool (strict)"(reference=w588) -> ("Value"=w579:bool)  [unwired: 1 in, 2 out]
            n183 = property class="Bool (strict)"(reference=w587) -> ("Value"=w580:bool)  [unwired: 1 in, 2 out]
            n184 = Index Array(array=w561) -> (element #1=w585:bool, element #2=w576:bool, element #3=w578:bool, element #4=w577:bool, element #5=w564:bool)  [unwired: 5 in]
            n185 = Not Equal?(x=w567, y=w562) -> (x != y?=w575:bool[])
            n186 = Boolean Array To Number(Boolean array=w575) -> (number=w573:u32)
            n187 = property class="Bool (strict)"(reference=w584, "Value"=w585) -> ()  [unwired: 1 in, 2 out]
            n188 = property class="Bool (strict)"(reference=w583) -> ("Value"=w563:bool)  [unwired: 1 in, 2 out]
            n189 = property class="Bool (strict)"(reference=w592) -> ("Value"=w565:bool)  [unwired: 1 in, 2 out]
            n190 = property class="Bool (strict)"(reference=w593) -> ("Value"=w566:bool)  [unwired: 1 in, 2 out]
            n191 = property class="Bool (strict)"(reference=w582) -> ("Value"=w581:bool)  [unwired: 1 in, 2 out]
            n192 = property class="Bool (strict)"(reference=w601, "Value"=w578) -> ()  [unwired: 1 in, 2 out]
            n193 = property class="Bool (strict)"(reference=w600, "Value"=w577) -> ()  [unwired: 1 in, 2 out]
            n194 = property class="Bool (strict)"(reference=w595) -> ("Value"=w591:bool)  [unwired: 1 in, 2 out]
            n195 = property class="Bool (strict)"(reference=w598) -> ("Value"=w590:bool)  [unwired: 1 in, 2 out]
            n196 = property class="Bool (strict)"(reference=w599, "Value"=w576) -> ()  [unwired: 1 in, 2 out]
            n197 = property class="Bool (strict)"(reference=w574, "Value"=w564) -> ()  [unwired: 1 in, 2 out]
            n198 = call "EvaluaParoEmergencia.vi"("EsticPujant"=w580, "FCI"=w577, "FCS"=w578, "EsticBaixant"=w579, "ParoManual"=w576) -> ("Paro"=w586:bool)  [unwired: 10 in]
            n199 = property on="ParoProcessat" class="Bool (strict)"() -> ("Value"=w597:bool)  [unwired: 2 in, 2 out]
            n200 = case shown="16" w573 {
              frame 0, Default {
              }
              frame 1 {
                n201 = property on="IniciAssaig" class="Bool (strict)"("Val(Sgnl)"=TRUE ("Value (Signaling)")) -> ()  [unwired: 2 in, 2 out]
              }
              frame 2 {
                n202 = property on="Paro Manual" class="Bool (strict)"("Val(Sgnl)"=TRUE ("Value (Signaling)")) -> ()  [unwired: 2 in, 2 out]
              }
              frame 4 {
                n203 = property on="FCS" class="Bool (strict)"("Val(Sgnl)"=TRUE ("Value (Signaling)")) -> ()  [unwired: 2 in, 2 out]
              }
              frame 8 {
                n204 = property on="FCI" class="Bool (strict)"("Val(Sgnl)"=TRUE ("Value (Signaling)")) -> ()  [unwired: 2 in, 2 out]
              }
              frame 16 {
                n205 = property on="Paro Emergencia" class="Bool (strict)"("Val(Sgnl)"=TRUE ("Value (Signaling)")) -> ()  [unwired: 2 in, 2 out]
              }
            }
            n206 = case shown="True" w586 {
              selector: w586 -> [w609 _]
              frame False {
                n207 = property on="ParoProcessat" class="Bool (strict)"("Value"=w609) -> ()  [unwired: 2 in, 2 out]
              }
              frame True {
              }
            }
            n208 = Not(x=w597) -> (.not. x?=w596:bool)
            n209 = And(x=w596, y=w586) -> (x .and. y?=w594:bool)
            n210 = Compound Arithmetic op=OR(w591, w594, w590) -> ()  [unwired: 1 out]
            n211 = case shown="True" w594 {
              selector: w594 -> [_ w618]
              tunnel: w591 -> [w612 w617]
              tunnel: w590 -> [w611 w616]
              tunnel: [w610 w614] -> w589
              frame False {
                n212 = Build Array(w612, w611) -> (w613:bool[])
                n213 = Boolean Array To Number(Boolean array=w613) -> (number=w610:u32)
              }
              frame True {
                n214 = Build Array(w617, w616) -> (w615:bool[])
                n215 = Boolean Array To Number(Boolean array=w615) -> (number=w614:u32)
                n216 = property on="Paro Emergencia" class="Bool (strict)"("Val(Sgnl)"=w618) -> ()  [unwired: 2 in, 2 out]
              }
            }
            "CodiAturada" <- w589
            n217 = Build Array(w566, w565, w581, w563) -> (w570:bool[])
          }
        }
        n218 = property on="Stop" class="Bool (strict)"() -> ("Value"=w534:bool)  [unwired: 2 in, 2 out]
        n219 = call-poly <vilib>:"DAQmx Write.vi"("task/channels in"=w514, "data"=w510, "error in"=w511) -> ("task out"=w513:refnum<k21>, "error out"=w512:errorcluster)  [unwired: 10 in, 1 out]
      }
      n220 = control-ref of="FactorsUnitatsPendents_D"() -> (w231:refnum<vi>)
      n221 = control-ref of="FactorsUnitatsPendents_F"() -> (w236:refnum<vi>)
      n222 = control-ref of="FactorsUnitatsTermesInp_D"() -> (w192:refnum<vi>)
      n223 = control-ref of="TaraF"() -> (w266:refnum<vi>)
      n224 = control-ref of="FSenseTara"() -> (w267:refnum<vi>)
      n225 = control-ref of="TablaFinal"() -> (w210:refnum<vi>)
      n226 = control-ref of="TaraD"() -> (w271:refnum<vi>)
      n227 = control-ref of="CaptadorF"() -> (w234:refnum<vi>)
      n228 = control-ref of="ParoProcessat"() -> (w223:refnum<vi>)
      n229 = control-ref of="NMostres"() -> (w213:refnum<vi>)
      n230 = while {
        shift-right: [w934] -> _
        shift-left: dbl[][] [] -> [w933]
        tunnel: w277 -> [w932]
        tunnel: w279 -> [w921]
        tunnel: w229 -> [w931]
        tunnel: w278 -> [w930]
        tunnel: w276 -> [w928]
        tunnel: [w929] -> w232
        tunnel: w275 -> [w927]
        tunnel: w274 -> [w926]
        tunnel: w272 -> [w925]
        tunnel: w273 -> [w924]
        tunnel: w269 -> [w923]
        tunnel: w268 -> [w922]
        shift-right: [w920] -> _
        shift-left: FALSE ("ControlaCaigudaSortida") -> [w919]
        tunnel: w265 -> [w918]
        tunnel: w257 -> [w917]
        tunnel: w235 -> [w916]
        tunnel: w233 -> [w915]
        tunnel: w217 -> [w913]
        tunnel: w214 -> [w911]
        tunnel: w210 -> [w910]
        tunnel: w193 -> [w909]
        tunnel: w192 -> [w908]
        stop <- w914 stop-if-true
        n231 = property on="Procesa datos" class="Bool (strict)"() -> ("Value"=w912:bool)  [unwired: 2 in, 2 out]
        n232 = property on="Ensayo activo" class="Bool (strict)"("Value"=w912) -> ()  [unwired: 2 in, 2 out]
        n233 = event shown="[0] <DadesAdquirides>: User Event" {
          selector: w928 -> [_ _ _ _]
          dyn-events: [_ _ _ _] -> w929
          timeout: _ -> [_ _ _ _]
          tunnel: w933 -> [w983 w1061 w1133 _]
          tunnel: [w982 w1060 w1132 _] -> w934
          tunnel: w912 -> [w942 w1062 _ _]
          tunnel: w932 -> [w976 _ _ _]
          tunnel: w921 -> [w977 _ _ _]
          tunnel: w931 -> [w948 _ _ _]
          tunnel: w930 -> [w978 _ _ _]
          tunnel: w927 -> [w980 _ _ _]
          tunnel: w926 -> [w958 _ _ _]
          tunnel: w925 -> [w970 _ _ _]
          tunnel: w924 -> [w979 _ _ _]
          tunnel: w923 -> [w950 _ w1129 _]
          tunnel: w922 -> [w964 _ w1130 _]
          tunnel: [w975 _ _ _] -> w920
          tunnel: w919 -> [w974 _ _ _]
          tunnel: w918 -> [w973 _ w1128 _]
          tunnel: w917 -> [w959 _ _ _]
          tunnel: w916 -> [w963 _ _ _]
          tunnel: w915 -> [_ _ _ _]
          tunnel: w913 -> [w944 _ _ _]
          tunnel: w911 -> [_ w1059 w1126 w1159]
          tunnel: w910 -> [_ _ w1127 _]
          tunnel: w909 -> [w937 _ _ _]
          tunnel: w908 -> [w936 _ _ _]
          event User Event {
            n234 = event-data() -> ("DadesAdquirides"=w956:dbl[])  [unwired: 1 in, 3 out]
            n235 = property on="Val. control sobrecarga" class="DigNum (strict)"() -> ("Value"=w961:dbl)  [unwired: 2 in, 2 out]
            n236 = Index Array(array=w956, index=0) -> (element=w943:dbl)
            n237 = call "ConverteixAD.vi"("ValorSenseTara"=w978, "ValorAdquirid"=w943, "FactorUnitatsTermesInd"=w937, "Unitats"=w964, "Tara"=w977, "FactorsUnitatsPendents"=w976) -> ("Escala"=w962:u8, "ValorActualAbs"=w972:dbl, "ValorSenseTara"=w969:dbl)  [unwired: 3 in]
            "ValorSenseTara" <- w969
            n238 = property on="CaptadorD" class="Ring (strict)"() -> ("Value"=w940:u16)  [unwired: 2 in, 2 out]
            n239 = Absolute Value(x=w969) -> (abs(x)=w946:dbl)
            n240 = property on="Sobrecarga" class="Bool (strict)"() -> ("Value"=w968:bool)  [unwired: 2 in, 2 out]
            n241 = Greater?(x=w946, y=w961) -> (0:w965:bool)
            n242 = case shown="0, Default" w940 {
              tunnel: [1 ("index") 2 ("index")] -> w952
              tunnel: w956 -> [w1005 w1006]
              tunnel: [w1005 w1006] -> w955
              frame 0, Default {
              }
              frame 1 {
              }
            }
            n243 = call "FormatDades.vi"("Captador"=w963, "Escala"=w962, "ValorIn"=w972, "Unidades"=w964) -> ("NDecimals"=w960:u8, "ValorOut"=w971:dbl)  [unwired: 6 in]
            n244 = Not(x=w968) -> (.not. x?=w966:bool)
            n245 = And(x=w965, y=w966) -> (x .and. y?=w967:bool)
            n246 = property on="BtMaxF" class="Bool (strict)"() -> ("Value"=w957:bool)  [unwired: 2 in, 2 out]
            n247 = Index Array(array=w955, index=w952) -> (element=w954:dbl)
            n248 = call "ConverteixAD.vi"("ValorSenseTara"=w979, "ValorAdquirid"=w954, "FactorUnitatsTermesInd"=w936, "Unitats"=w950, "Tara"=w970, "FactorsUnitatsPendents"=w980) -> ("ValorActualAbs"=w941:dbl)  [unwired: 3 in, 2 out]
            n249 = case shown="True" w967 {
              selector: w967 -> [_ w1056]
              tunnel: w965 -> [w1055 _]
              frame False {
                n250 = property on="Sobrecarga" class="Bool (strict)"("Value"=w1055) -> ()  [unwired: 2 in, 2 out]
              }
              frame True {
                n251 = property on="Sobrecarga" class="Bool (strict)"("Val(Sgnl)"=w1056) -> ()  [unwired: 2 in, 2 out]
              }
            }
            n252 = case shown="True" w957 {
              tunnel: w948 -> [w1012 w1016]
              tunnel: w971 -> [w1011 w1013]
              tunnel: w960 -> [w1010 w1018]
              tunnel: w959 -> [_ w1017]
              tunnel: [w1009 w1015] -> w947
              tunnel: [w1008 w1013] -> w945
              frame False {
                n253 = property class="DigNum (strict)"(reference=w1012, "Value"=w1011, "Precision"=w1010) -> (error out=w1009:errorcluster, "Value"=w1008:sgl)  [unwired: 1 in, 1 out]
              }
              frame True {
                n254 = property class="DigNum (strict)"(reference=w1017) -> (error out=w1019:errorcluster, "Value"=w1014:sgl)  [unwired: 1 in, 1 out]
                n255 = property class="DigNum (strict)"(reference=w1016, error in=w1019, "Value"=w1014, "Precision"=w1018) -> (error out=w1015:errorcluster)  [unwired: 1 out]
              }
            }
            n256 = property on="ResoExten" class="Ring (strict)"() -> ("Value"=w935:i8)  [unwired: 2 in, 2 out]
            n257 = property on="UnidadesD" class="Ring (strict)"() -> ("Value"=w949:u16)  [unwired: 2 in, 2 out]
            n258 = case shown="0, Default" w940 {
              selector: w940 -> [w995 w998]
              tunnel: [w994 w1003] -> w953
              tunnel: [u8 1 ("NDecimals") w1000] -> w951
              tunnel: w941 -> [w994 w1002]
              tunnel: w940 -> [_ _]
              tunnel: w949 -> [w997 w1001]
              tunnel: w935 -> [w996 w999]
              frame 0, Default {
                n259 = call "FormatDefor.vi"("UnidadesD"=w997, "ValorIn"=w994, "CaptadorD"=w995, "ResoExten"=w996) -> ()  [unwired: 6 in, 2 out]
              }
              frame 1 {
                n260 = call "FormatDefor.vi"("UnidadesD"=w1001, "ValorIn"=w1002, "CaptadorD"=w998, "ResoExten"=w999) -> ("ValorOut"=w1003:dbl, "NDecimals"=w1000:u8)  [unwired: 6 in]
              }
            }
            n261 = case shown="False" "BtMaxD" {
              tunnel: w958 -> [w987 w988]
              tunnel: w953 -> [w986 w992]
              tunnel: w951 -> [w985 w991]
              tunnel: [w984 w992] -> w939
              frame False {
                n262 = property class="DigNum (strict)"(reference=w987, "Value"=w986, "Precision"=w985) -> ("Value"=w984:sgl)  [unwired: 1 in, 2 out]
              }
              frame True {
                n263 = property on="MaximDaFmax" class="DigNum (strict)"() -> (error out=w990:errorcluster, "Value"=w989:sgl)  [unwired: 2 in, 1 out]
                n264 = property class="DigNum (strict)"(reference=w988, error in=w990, "Value"=w989, "Precision"=w991) -> ()  [unwired: 2 out]
              }
            }
            n265 = case shown="True" w942 {
              tunnel: w983 -> [_ w1050]
              tunnel: [_ w1049] -> w982
              tunnel: [FALSE ("ControlaCaigudaSortida") w1047] -> w975
              tunnel: w974 -> [_ w1051]
              tunnel: w973 -> [_ w1052]
              tunnel: w959 -> [_ w1048]
              tunnel: w947 -> [_ _]
              tunnel: w945 -> [_ w1027]
              tunnel: w944 -> [_ w1046]
              tunnel: w939 -> [_ w1023]
              frame False {
                n266 = property on="ParaAssaig" class="Bool (strict)"("Value"=FALSE ("ParaAssaig")) -> ()  [unwired: 2 in, 2 out]
                n267 = property on="ParoRotura" class="Bool (strict)"("Value"=FALSE ("ParoRotura")) -> ()  [unwired: 2 in, 2 out]
              }
              frame True {
                w1041 = 0
                n268 = property on="Valor de control Paro Rotura" class="DigNum (strict)"() -> ("Value"=w1026:dbl)  [unwired: 2 in, 2 out]
                n269 = property class="DigNum (strict)"(reference=w1052) -> ("Value"=w1038:sgl)  [unwired: 1 in, 2 out]
                n270 = property class="DigNum (strict)"(reference=w1048) -> (reference out=w1035:refnum<vi>, "Value"=w1036:sgl)  [unwired: 1 in, 1 out]
                n271 = Greater?(x=w1027, y=w1026) -> (0:w1025:bool)
                n272 = property class="DigNum (strict)"(reference=w1046) -> (reference out=w1030:refnum<vi>, "Value"=w1032:dbl)  [unwired: 1 in, 1 out]
                n273 = call "ControlFiAssaig.vi"("Actiu"=w1025, "PercentatgeCaiguda"=w1038, "ControlaCaigudaEntrada"=w1051, "ValorActual"=w1027, "ValorMaxim"=w1036) -> (0:"NouMaxim"=w1024:bool, "ControlaCaigudaSortida"=w1047:bool, "ParoRotura"=w1033:bool, 3:"NouMaxim"=w1034:dbl)  [unwired: 3 in]
                n274 = Increment(x=w1032) -> (x+1=w1031:dbl)
                n275 = case shown="True" w1024 {
                  tunnel: w1023 -> [_ w1053]
                  frame False {
                  }
                  frame True {
                    n276 = property on="MaximDaFmax" class="DigNum (strict)"("Value"=w1053) -> ()  [unwired: 2 in, 2 out]
                  }
                }
                n277 = property class="DigNum (strict)"(reference=w1030, "Value"=w1031) -> ()  [unwired: 1 in, 2 out]
                n278 = property class="DigNum (strict)"(reference=w1035, "Value"=w1034) -> ()  [unwired: 1 in, 2 out]
                n279 = Array Size(array=w1050) -> (size(s)=w1042:i32[])
                n280 = Index Array(array=w1042, index=w1041) -> (element=w1040:i32)
                n281 = property on="ActivaParoRotura" class="Bool (strict)"() -> ("Value"=w1028:bool)  [unwired: 2 in, 2 out]
                n282 = Equal?(x=w1040, y=w1041) -> (x = y?=w1039:bool)
                n283 = And(x=w1028, y=w1033) -> (x .and. y?=w1029:bool)
                n284 = Merge Signals(w1023, w1027) -> (w1043:dynamicdata)
                n285 = call "Build XY Graph"("Reset"=w1039, "Y Input"=w1027, "X Input"=w1023) -> ("XY Graph"=→"?":cluster{"Y":dbl[], "Y":dbl[]}[])  [unwired: 7 in, 1 out]
                n286 = case shown="True" w1029 {
                  selector: w1029 -> [_ w1054]
                  frame False {
                  }
                  frame True {
                    n287 = property on="ParoRotura" class="Bool (strict)"("Val(Sgnl)"=w1054) -> ()  [unwired: 2 in, 2 out]
                  }
                }
                n288 = property on="First time" class="Bool (strict)"("Value"=TRUE) -> ()  [unwired: 2 in, 2 out]
                n289 = call "Convert from Dynamic Data"("Dynamic Data Type"=w1043) -> ("Array"=w1037:dbl[])  [unwired: 3 in]
                n290 = Build Array (concatenate)(w1050, w1037) -> (w1049:dbl[][])
                "Tabla" <- w1049
              }
            }
          }
          event "Salir": Value Change {
            n291 = event-data() -> ()  [unwired: 1 in, 6 out]
            n292 = property on="rings" class="Arr (strict)"() -> ("Value"=w1058:refnum<vi>[])  [unwired: 2 in, 2 out]
            n293 = property on="Caselles" class="Arr (strict)"() -> ("Value"=w1057:refnum<vi>[])  [unwired: 2 in, 2 out]
            n294 = case shown="False" w1062 {
              selector: w1062 -> [_ w1097]
              tunnel: w1061 -> [_ w1099]
              tunnel: [_ w1099] -> w1060
              tunnel: w1059 -> [_ w1096]
              tunnel: w1058 -> [w1067 w1093]
              tunnel: w1057 -> [w1066 w1092]
              frame False {
                n295 = flat-sequence {
                  tunnel: w1067 -> [w1070]
                  tunnel: w1066 -> [w1069]
                  tunnel: [w1068] -> w1065
                  tunnel: [w1072] -> w1064
                  tunnel: w1065 -> [w1072]
                  tunnel: w1064 -> [w1085]
                  tunnel: [w1085] -> w1063
                  tunnel: w1063 -> [w1087]
                  frame #0 {
                    n296 = call "GuardaValorsPantalla.vi"("Rings"=w1070, "Caselles"=w1069) -> ("error out"=w1068:errorcluster)  [unwired: 8 in]
                  }
                  frame #1 {
                    n297 = call <vilib>:"DAQmx Stop Task.vi"("task/channels in"=refnum<k21> "Esclatometre_USBAnalogIn") -> ("task out"=w1081:refnum<k21>, "error out"=w1080:errorcluster)  [unwired: 13 in]
                    n298 = call <vilib>:"DAQmx Stop Task.vi"("task/channels in"=refnum<k21> "Esclatometre_USBAnalogOut") -> ("task out"=w1076:refnum<k21>, "error out"=w1078:errorcluster)  [unwired: 13 in]
                    n299 = call <vilib>:"DAQmx Stop Task.vi"("task/channels in"=refnum<k21> "Esclatometre_USBSDigitalIn") -> ("task out"=w1074:refnum<k21>, "error out"=w1075:errorcluster)  [unwired: 13 in]
                    n300 = call <vilib>:"DAQmx Stop Task.vi"("task/channels in"=refnum<k21> "Esclatometre_USBDigitalOut") -> ("task out"=w1083:refnum<k21>, "error out"=w1082:errorcluster)  [unwired: 13 in]
                    n301 = call <vilib>:"DAQmx Clear Task.vi"("task in"=w1081, "error in"=w1080) -> ()  [unwired: 13 in, 1 out]
                    n302 = call <vilib>:"DAQmx Clear Task.vi"("task in"=w1076, "error in"=w1078) -> ()  [unwired: 13 in, 1 out]
                    n303 = call <vilib>:"DAQmx Clear Task.vi"("task in"=w1074, "error in"=w1075) -> ()  [unwired: 13 in, 1 out]
                    n304 = call <vilib>:"DAQmx Clear Task.vi"("task in"=w1083, "error in"=w1082) -> ()  [unwired: 13 in, 1 out]
                  }
                  frame #2 {
                    n305 = Wait (ms)(milliseconds to wait=u32 500) -> ()  [unwired: 1 out]
                  }
                  frame #3 {
                    (unwired) TRUE
                    n306 = property on="Calibrar" class="Bool (strict)"() -> ("Value"=w1086:bool)  [unwired: 2 in, 2 out]
                    n307 = case shown="False" w1086 {
                      tunnel: w1087 -> [w1088 _]
                      frame False {
                        n308 = disable-structure shown="RUN_TIME_ENGINE==True" {
                          disable-tunnel: w1088 -> [_ _]
                          frame condition #0 (active) {
                            n309 = Quit LabVIEW(quit? (T)=errorcluster {"status"=TRUE, "code"=0, "source"=""}) -> ()
                          }
                          frame condition #1 {
                            n310 = call <vilib>:"System Exec.vi"("command line"="cmd.exe /C shutdown -s -t 0") -> ()  [unwired: 7 in, 4 out]
                          }
                        }
                      }
                      frame True {
                        n311 = Quit LabVIEW(quit? (T)=errorcluster {"status"=TRUE, "code"=0, "source"=""}) -> ()
                      }
                    }
                  }
                }
              }
              frame True {
                # "Mensaje de cancelar o no el ensayo activo"
                n312 = Index Array(array=w1096, index=2) -> (element=w1094:string)
                n313 = call "Display Message to User2"("Enable"=w1097, "Message"=w1094) -> ("OK"=w1098:bool)  [unwired: 8 in, 1 out]
                n314 = case shown="True" w1098 {
                  tunnel: w1093 -> [_ w1105]
                  tunnel: w1092 -> [_ w1104]
                  frame False {
                    n315 = property on="Salir" class="Bool (strict)"("Value"=FALSE ("Salir")) -> ()  [unwired: 2 in, 2 out]
                  }
                  frame True {
                    n316 = flat-sequence {
                      tunnel: w1105 -> [w1108]
                      tunnel: w1104 -> [w1107]
                      tunnel: [w1106] -> w1103
                      tunnel: [w1109] -> w1102
                      tunnel: w1103 -> [w1109]
                      tunnel: w1102 -> [w1123]
                      tunnel: [w1123] -> w1101
                      tunnel: w1101 -> [w1124]
                      frame #0 {
                        n317 = call "GuardaValorsPantalla.vi"("Rings"=w1108, "Caselles"=w1107) -> ("error out"=w1106:errorcluster)  [unwired: 8 in]
                      }
                      frame #1 {
                        n318 = call <vilib>:"DAQmx Stop Task.vi"("task/channels in"=refnum<k21> "Esclatometre_USBAnalogIn") -> ("task out"=w1119:refnum<k21>, "error out"=w1118:errorcluster)  [unwired: 13 in]
                        n319 = call <vilib>:"DAQmx Stop Task.vi"("task/channels in"=refnum<k21> "Esclatometre_USBAnalogOut") -> ("task out"=w1114:refnum<k21>, "error out"=w1116:errorcluster)  [unwired: 13 in]
                        n320 = call <vilib>:"DAQmx Stop Task.vi"("task/channels in"=refnum<k21> "Esclatometre_USBDigitalOut") -> ("task out"=w1121:refnum<k21>, "error out"=w1120:errorcluster)  [unwired: 13 in]
                        n321 = call <vilib>:"DAQmx Stop Task.vi"("task/channels in"=refnum<k21> "Esclatometre_USBDigitalOut") -> ("task out"=w1112:refnum<k21>, "error out"=w1113:errorcluster)  [unwired: 13 in]
                        n322 = call <vilib>:"DAQmx Clear Task.vi"("task in"=w1121, "error in"=w1120) -> ()  [unwired: 13 in, 1 out]
                        n323 = call <vilib>:"DAQmx Clear Task.vi"("task in"=w1119, "error in"=w1118) -> ()  [unwired: 13 in, 1 out]
                        n324 = call <vilib>:"DAQmx Clear Task.vi"("task in"=w1114, "error in"=w1116) -> ()  [unwired: 13 in, 1 out]
                        n325 = call <vilib>:"DAQmx Clear Task.vi"("task in"=w1112, "error in"=w1113) -> ()  [unwired: 13 in, 1 out]
                      }
                      frame #2 {
                        n326 = Wait (ms)(milliseconds to wait=u32 500) -> ()  [unwired: 1 out]
                      }
                      frame #3 {
                        n327 = disable-structure shown="RUN_TIME_ENGINE==True" {
                          disable-tunnel: w1124 -> [_ _]
                          frame condition #0 (active) {
                          }
                          frame condition #1 {
                            n328 = call <vilib>:"System Exec.vi"("command line"="cmd.exe /C shutdown -s -t 0") -> ()  [unwired: 7 in, 4 out]
                          }
                        }
                      }
                    }
                  }
                }
              }
            }
          }
          event "Guardar": Value Change {
            n329 = event-data() -> ("NewVal"=w1131:bool)  [unwired: 1 in, 5 out]
            n330 = case shown="True" w1131 {
              tunnel: w1133 -> [w1134 w1136]
              tunnel: [w1134 w1136] -> w1132
              tunnel: w1130 -> [_ _]
              tunnel: w1129 -> [_ _]
              tunnel: w1128 -> [_ _]
              tunnel: w1127 -> [_ _]
              tunnel: w1126 -> [_ w1135]
              frame False {
              }
              frame True {
                n331 = flat-sequence {
                  tunnel: w1135 -> [w1138]
                  frame #0 {
                    n332 = property on="Nº Tests" class="DigNum (strict)"() -> ("Value"=w1140:u8)  [unwired: 2 in, 2 out]
                    n333 = property on="Guardar" class="Bool (strict)"("Value"=FALSE) -> ()  [unwired: 2 in, 2 out]
                    n334 = Greater Than 0?(x=w1140) -> (x > 0?=w1139:bool)
                    n335 = case shown="True" w1139 {
                      tunnel: w1138 -> [w1143 _]
                      frame False {
                        n336 = Index Array(array=w1143, index=6) -> (element=w1141:string)
                        n337 = call "Display Message to User4"("Message"=w1141) -> ()  [unwired: 9 in, 2 out]
                      }
                      frame True {
                        n338 = property on="ArraiMaxF_D" class="Arr (strict)"() -> ("Value"=w1147:dbl[][])  [unwired: 2 in, 2 out]
                        n339 = call <vilib>:"Application Directory.vi"() -> ("Application Directory"=w1155:path)
                        n340 = Transpose 2D Array(2D array=w1147) -> (transposed array=w1146:dbl[][])
                        n341 = Build Path(base path=w1155, name or relative path="Datos") -> (appended path=w1149:path)
                        n342 = Build Path(base path=w1149, name or relative path="Lectura.txt" ("string")) -> (appended path=w1148:path)
                        n343 = call-poly <vilib>:"Write Delimited Spreadsheet.vi"("file path (dialog if empty)"=w1148, "2D data"=w1146, "append to file? (new file:F)"=FALSE, "transpose? (no:F)"=TRUE, "delimiter (\\t)"=";" ("delimiter (\\t)")) -> ("error out"=w1151:errorcluster)  [unwired: 9 in, 1 out]
                        n344 = case shown="No Error" w1151 {
                          tunnel: ["Informe generado con éxito" ("Message") "Error generando informe" ("Message")] -> w1144
                          frame No Error {
                          }
                          frame Error {
                          }
                        }
                        n345 = property on="Estado ensayo:" class="Str"("Value"=w1144) -> ()  [unwired: 2 in, 2 out]
                      }
                    }
                  }
                  frame #1 {
                    n346 = property on="Ensayonuevo" class="Bool (strict)"("Val(Sgnl)"=TRUE ("Value (Signaling)")) -> ()  [unwired: 2 in, 2 out]
                  }
                }
              }
            }
          }
          event "BtEliminarUltima": Value Change {
            n347 = event-data() -> ("NewVal"=w1160:bool)  [unwired: 1 in, 5 out]
            n348 = case shown="True" w1160 {
              tunnel: w1159 -> [_ w1161]
              frame False {
              }
              frame True {
                n349 = property on="Nº Tests" class="DigNum (strict)"() -> ("Value"=w1162:u8)  [unwired: 2 in, 2 out]
                n350 = Greater Than 0?(x=w1162) -> (x > 0?=w1163:bool)
                n351 = case shown="True" w1163 {
                  tunnel: w1162 -> [_ w1171]
                  tunnel: w1161 -> [w1166 w1169]
                  frame False {
                    n352 = Index Array(array=w1166, index=4) -> (element=w1164:string)
                    n353 = call "Display Message to User3"("Message"=w1164) -> ()  [unwired: 9 in, 2 out]
                  }
                  frame True {
                    n354 = Index Array(array=w1169, index=3) -> (element=w1167:string)
                    n355 = call "Display Message to User6"("Message"=w1167) -> ("OK"=w1170:bool)  [unwired: 9 in, 1 out]
                    n356 = case shown="True" w1170 {
                      tunnel: w1171 -> [_ w1179]
                      frame False {
                      }
                      frame True {
                        w1182 = u8 2 ("y")
                        n357 = Subtract(x=w1179, y=1.0) -> (x-y=w1181:dbl)
                        n358 = Multiply(x=w1179, y=w1182) -> (x*y=w1183:u8)
                        n359 = property on="TablaFinal" class="Arr (strict)"() -> ("Value"=w1175:dbl[][])  [unwired: 2 in, 2 out]
                        n360 = property on="Nº Tests" class="DigNum (strict)"("Value"=w1181) -> ()  [unwired: 2 in, 2 out]
                        n361 = Subtract(x=w1183, y=w1182) -> (x-y=w1173:u8)
                        n362 = property on="Columna" class="DigNum (strict)"("Value"=w1173) -> ()  [unwired: 2 in, 2 out]
                        n363 = Initialize Array(0.0 ("element"), 3600 ("dimension size"), 2 ("dimension size")) -> ()  [unwired: 1 out]
                        n364 = Delete From Array(array=w1175, length=3600, index (col)=w1173) -> (array with subset deleted=w1174:dbl[][])  [unwired: 1 in, 1 out]
                        n365 = property on="TablaFinal" class="Arr (strict)"("Value"=w1174) -> ()  [unwired: 2 in, 2 out]
                      }
                    }
                  }
                }
              }
            }
          }
        }
        n366 = property on="Stop" class="Bool (strict)"() -> ("Value"=w914:bool)  [unwired: 2 in, 2 out]
      }
      n367 = control-ref of="Tabla"() -> (w211:refnum<vi>)
      n368 = control-ref of="Maxim"() -> (w200:refnum<vi>)
      n369 = control-ref of="ArraiMaxims"() -> (w199:refnum<vi>)
      n370 = control-ref of="TablaFinal"() -> (w212:refnum<vi>)
      n371 = control-ref of="ArraiMaxF_D"() -> (w194:refnum<vi>)
      n372 = while {
        tunnel: w270 -> [w721]
        tunnel: w271 -> [w720]
        tunnel: w267 -> [w719]
        tunnel: w266 -> [w718]
        tunnel: w236 -> [w717]
        tunnel: w234 -> [w716]
        tunnel: w231 -> [w715]
        tunnel: w223 -> [w714]
        tunnel: w214 -> [w713]
        tunnel: w213 -> [w712]
        tunnel: w212 -> [w711]
        tunnel: w211 -> [w710]
        tunnel: w200 -> [w709]
        tunnel: w199 -> [w708]
        tunnel: w194 -> [w707]
        stop <- w722 stop-if-true
        n373 = event shown="[0] \"Iniciar / Finalizar\": Value Change" {
          selector: _ -> [_ _ _ _ _ _ _ _ _]
          dyn-events: _ -> [_ _ _ _ _ _ _ _ _]
          timeout: _ -> [_ _ _ _ _ _ _ _ _]
          tunnel: w721 -> [w725 _ _ _ _ _ _ w904 _]
          tunnel: w720 -> [w724 _ _ w842 _ _ _ w901 _]
          tunnel: w719 -> [_ _ _ _ _ _ _ _ w907]
          tunnel: w718 -> [_ _ w826 _ _ _ _ _ w906]
          tunnel: [_ _ _ _ w849 w880 _ _ _] -> _
          tunnel: w717 -> [_ _ _ _ w849 w880 _ _ _]
          tunnel: w716 -> [_ _ w827 _ w845 _ _ _ _]
          tunnel: w715 -> [_ _ _ _ _ w879 _ _ _]
          tunnel: [_ _ _ _ _ _ _ w904 _] -> _
          tunnel: w714 -> [_ _ _ _ _ _ w886 _ _]
          tunnel: w713 -> [w732 w800 _ _ _ _ _ _ _]
          tunnel: w712 -> [w731 _ _ _ _ _ _ _ _]
          tunnel: w711 -> [w730 w799 _ _ _ _ _ _ _]
          tunnel: w710 -> [w729 _ _ _ _ _ _ _ _]
          tunnel: w709 -> [w726 _ _ _ _ _ _ _ _]
          tunnel: w708 -> [_ w798 _ _ _ _ _ _ _]
          tunnel: w707 -> [w723 w797 _ _ _ _ _ _ _]
          event "Iniciar / Finalizar": Value Change {
            n374 = event-data() -> ()  [unwired: 1 in, 5 out]
            n375 = property on="IniciAssaig" class="Bool (strict)"() -> ("Value"=w727:bool)  [unwired: 2 in, 2 out]
            n376 = property on="Iniciar / Finalizar" class="Bool (strict)"() -> ("Value"=w733:bool)  [unwired: 2 in, 2 out]
            n377 = Or(x=w733, y=w727) -> (x .or. y?=w728:bool)
            n378 = case shown="True" w728 {
              tunnel: w732 -> [_ w793]
              tunnel: w731 -> [w740 _]
              tunnel: w730 -> [w737 _]
              tunnel: w729 -> [w736 _]
              tunnel: w726 -> [w735 _]
              tunnel: w725 -> [_ w788]
              tunnel: w724 -> [_ w787]
              tunnel: w723 -> [w734 _]
              frame False {
                n379 = flat-sequence {
                  tunnel: w740 -> [w747]
                  tunnel: [w745] -> w738
                  tunnel: w737 -> [w744]
                  tunnel: w736 -> [w743]
                  tunnel: w735 -> [w742]
                  tunnel: w734 -> [w741]
                  tunnel: [w780] -> w739
                  tunnel: w738 -> [w780]
                  tunnel: w739 -> [w783]
                  frame #0 {
                    n380 = property on="Procesa datos" class="Bool (strict)"("Value"=FALSE) -> ()  [unwired: 2 in, 2 out]
                    n381 = property on="ParaAssaig" class="Bool (strict)"("Value"=TRUE ("ParaAssaig")) -> ()  [unwired: 2 in, 2 out]
                    n382 = property on="First time" class="Bool (strict)"() -> ("Value"=w746:bool)  [unwired: 2 in, 2 out]
                    n383 = case shown="True" w746 {
                      tunnel: w747 -> [w750 w770]
                      tunnel: [w750 w768] -> w745
                      tunnel: w744 -> [_ w767]
                      tunnel: w743 -> [_ w763]
                      tunnel: w742 -> [_ w761]
                      tunnel: w741 -> [_ w758]
                      frame False {
                      }
                      frame True {
                        n384 = property class="DigNum (strict)"(reference=w770) -> (reference out=w768:refnum<vi>, "Value"=w769:dbl)  [unwired: 1 in, 1 out]
                        n385 = property class="DigNum (strict)"(reference=w761) -> ("Value"=w755:sgl)  [unwired: 1 in, 2 out]
                        n386 = property on="Nº Tests" class="DigNum (strict)"() -> ("Value"=w756:u8)  [unwired: 2 in, 2 out]
                        n387 = property class="Arr (strict)"(reference=w758) -> (reference out=w752:refnum<vi>, "Value"=w757:dbl[][])  [unwired: 1 in, 1 out]
                        n388 = Increment(x=w756) -> (x+1=w776:u8)
                        n389 = property on="Nº Tests" class="DigNum (strict)"("Value"=w776) -> ()  [unwired: 2 in, 2 out]
                        n390 = property on="ArraiMostresxProva" class="Arr (strict)"() -> ("Value"=w775:dbl[])  [unwired: 2 in, 2 out]
                        n391 = property on="MaximDaFmax" class="DigNum (strict)"() -> ("Value"=w753:sgl)  [unwired: 2 in, 2 out]
                        n392 = property on="ArraiMaxims" class="Arr (strict)"() -> ("Value"=w760:sgl[])  [unwired: 2 in, 2 out]
                        n393 = Insert Into Array(array=w775, index=w756, new element=w769) -> (w774:dbl[])
                        n394 = Build Array(w755, w753) -> (w754:sgl[])
                        n395 = property on="ArraiMostresxProva" class="Arr (strict)"("Value"=w774) -> ()  [unwired: 2 in, 2 out]
                        n396 = Insert Into Array(array=w760, index=w756, new element=w755) -> (w759:sgl[])
                        n397 = Insert Into Array(array=w757, index (row)=w756, new element=w754) -> (w751:dbl[][])  [unwired: 1 in]
                        n398 = property class="Arr (strict)"(reference=w763) -> ("Value"=w762:dbl[][])  [unwired: 1 in, 2 out]
                        n399 = property on="ArraiMaxims" class="Arr (strict)"("Value"=w759) -> ()  [unwired: 2 in, 2 out]
                        n400 = property class="Arr (strict)"(reference=w767) -> (reference out=w765:refnum<vi>, "Value"=w766:dbl[][])  [unwired: 1 in, 1 out]
                        n401 = property class="Arr (strict)"(reference=w752, "Value"=w751) -> ()  [unwired: 1 in, 2 out]
                        n402 = property on="Columna" class="DigNum (strict)"() -> ("Value"=w777:i32)  [unwired: 2 in, 2 out]
                        n403 = property on="CodiAturada" class="DigNum (strict)"() -> ("Value"=w771:u32)  [unwired: 2 in, 2 out]
                        n404 = property on="StringsEstatMáquina" class="Arr (strict)"() -> ("Value"=w773:string[])  [unwired: 2 in, 2 out]
                        n405 = Insert Into Array(array=w766, index (col)=w777, new element=w762) -> (w764:dbl[][])  [unwired: 1 in]
                        n406 = Index Array(array=w773, index=w771) -> (element=w772:string)
                        n407 = property class="Arr (strict)"(reference=w765, "Value"=w764) -> ()  [unwired: 1 in, 2 out]
                        n408 = Add(x=w777, y=2) -> (x+y=w778:i32)
                        n409 = property on="Estado ensayo:" class="Str"("Value"=w772) -> ()  [unwired: 2 in, 2 out]
                        n410 = property on="Columna" class="DigNum (strict)"("Value"=w778) -> ()  [unwired: 2 in, 2 out]
                      }
                    }
                  }
                  frame #1 {
                    n411 = Wait (ms)(milliseconds to wait=u32 200) -> ()  [unwired: 1 out]
                  }
                  frame #2 {
                    n412 = property class="DigNum (strict)"(reference=w783, "Value"=0.0 ("NMostres")) -> ()  [unwired: 1 in, 2 out]
                    n413 = property on="First time" class="Bool (strict)"("Value"=FALSE) -> ()  [unwired: 2 in, 2 out]
                    n414 = property on="Tabla" class="Arr (strict)"("Value"=dbl[][] [] ("Tabla")) -> ()  [unwired: 2 in, 2 out]
                    n415 = property on="Rep. Fetes" class="DigNum (strict)"("Value"=u8 0 ("Rep. Fetes")) -> ()  [unwired: 2 in, 2 out]
                  }
                  frame #3 {
                  }
                }
              }
              frame True {
                n416 = property class="DigNum (strict)"(reference=w788) -> (error out=w790:errorcluster, "Value"=w789:sgl)  [unwired: 1 in, 1 out]
                n417 = Index Array(array=w793, index=18) -> (element=w792:string)
                n418 = property on="Estado ensayo:" class="Str"("Value"=w792) -> ()  [unwired: 2 in, 2 out]
                n419 = property class="DigNum (strict)"(reference=w787, error in=w790, "Value"=w789) -> ()  [unwired: 2 out]
                n420 = property on="Maxim" class="DigNum (strict)"("Value"=0.0 ("Maxim")) -> (error out=w794:errorcluster)  [unwired: 2 in, 1 out]
                n421 = property on="Procesa datos" class="Bool (strict)"(error in=w794, "Value"=TRUE) -> ()  [unwired: 1 in, 2 out]
              }
            }
          }
          event "Ensayonuevo": Value Change {
            n422 = event-data() -> ("NewVal"=w801:bool)  [unwired: 1 in, 5 out]
            n423 = case shown="True" w801 {
              tunnel: w800 -> [_ _]
              tunnel: [_ w812] -> _
              tunnel: w799 -> [_ w812]
              tunnel: w798 -> [_ w811]
              tunnel: w797 -> [_ w810]
              frame False {
              }
              frame True {
                n424 = property on="Columna" class="DigNum (strict)"("Value"=0 ("Columna")) -> ()  [unwired: 2 in, 2 out]
                n425 = Initialize Array(0.0 ("element"), 3600 ("dimension size"), 2 ("dimension size")) -> (w804:dbl[][])
                n426 = property class="Arr (strict)"(reference=w811, "Value"=sgl[] []) -> ()  [unwired: 1 in, 2 out]
                n427 = property class="Arr (strict)"(reference=w810, "Value"=dbl[][] []) -> ()  [unwired: 1 in, 2 out]
                n428 = property on="Nº Tests" class="DigNum (strict)"("Value"=u8 0 ("Nº Tests")) -> ()  [unwired: 2 in, 2 out]
                n429 = property class="Arr (strict)"(reference=w812, "Value"=w804) -> ()  [unwired: 1 in, 2 out]
              }
            }
          }
          event "UnidadesF": Value Change {
            n430 = event-data() -> ("NewVal"=w817:u16)  [unwired: 1 in, 5 out]
            n431 = property class="Ring (strict)"(reference=w827) -> ("Strings []"=w815:string[], "RingText.Text"=w814:string)  [unwired: 1 in, 2 out]
            n432 = Search 1D Array(1D array=w815, element=w814) -> (index of element=w816:i32)  [unwired: 1 in]
            n433 = property on="ConversioUnitatsF" class="Arr (strict)"() -> ("Value"=w828:dbl[])  [unwired: 2 in, 2 out]
            n434 = property class="DigNum (strict)"(reference=w826, "Value"=sgl 0.0) -> ()  [unwired: 1 in, 2 out]
            n435 = case shown="0, Default" w816 {
              tunnel: [w830 w831] -> w824
              frame 0, Default {
                n436 = property on="ValorSobrecargaC1" class="DigNum (strict)"() -> ("Value"=w830:dbl)  [unwired: 2 in, 2 out]
              }
              frame 1 {
                n437 = property on="ValorSobrecargaC2" class="DigNum (strict)"() -> ("Value"=w831:dbl)  [unwired: 2 in, 2 out]
              }
            }
            n438 = property on="UnidadesF" class="Ring (strict)"("Value"=w817) -> ()  [unwired: 2 in, 2 out]
            n439 = Index Array(array=w828, index=w817) -> (element=w829:dbl)
            n440 = Multiply(x=w824, y=w829) -> (x*y=w823:dbl)
            n441 = property on="Valor de control sobrecarga" class="DigNum (strict)"("Value"=w823) -> ()  [unwired: 2 in, 2 out]
            n442 = property on="ArraiUnitats" class="Arr (strict)"() -> ("Value"=w822:cluster{"String":string, "Value":u16}[])  [unwired: 2 in, 2 out]
            n443 = Index Array(array=w822, index=w817) -> (element=w821:cluster{"String":string, "Value":u16})
            n444 = Unbundle By Name(w821) -> ("String"=w818:string)
            n445 = property on="Fuerza" class="DigNum (strict)"() -> ("Caption.Text"=w813:string)  [unwired: 2 in, 2 out]
            n446 = Concatenate Strings(w813, " - " ("string"), w818) -> (w820:string)
            n447 = property class="XYGraph (strict)"("YScale.NameLbl.Text"=w820) -> ()  [unwired: 2 in, 2 out]
          }
          event "UnidadesD": Value Change {
            n448 = event-data() -> ("NewVal"=w837:u16)  [unwired: 1 in, 5 out]
            n449 = property class="DigNum (strict)"(reference=w842, "Value"=sgl 0.0) -> ()  [unwired: 1 in, 2 out]
            n450 = property on="UnidadesD" class="Ring (strict)"() -> ("StringsAndValues[]"=w838:T6)  [unwired: 2 in, 2 out]
            n451 = property class="XYGraph (strict)"() -> ("XScale.NameLbl.Text"=w840:string)  [unwired: 2 in, 2 out]
            n452 = Index Array(array=w838, index=w837) -> (element=w835:cluster{"String":string, "Value":u16})
            n453 = Unbundle By Name(w835) -> ("String"=w833:string)
            n454 = Match Pattern(string=w840, regular expression="-") -> (before substring=w836:string)  [unwired: 1 in, 3 out]
            n455 = Concatenate Strings(w836, "- " ("regular expression"), w833) -> (w834:string)
            n456 = property class="XYGraph (strict)"("XScale.NameLbl.Text"=w834) -> ()  [unwired: 2 in, 2 out]
          }
          event "CaptadorF": Value Change {
            n457 = event-data() -> ()  [unwired: 1 in, 6 out]
            n458 = property class="Ring (strict)"(reference=w845) -> ("Strings []"=w847:string[], "RingText.Text"=w846:string)  [unwired: 1 in, 2 out]
            n459 = Search 1D Array(1D array=w847, element=w846) -> (index of element=w844:i32)  [unwired: 1 in]
            n460 = Equal?(x=w844, y=0) -> (x = y?=w848:bool)
            n461 = flat-sequence {
              tunnel: w849 -> [w857]
              tunnel: w848 -> [w856]
              frame #0 {
                n462 = case shown="True" w856 {
                  tunnel: [w863 w865] -> w853
                  tunnel: [w864 w867] -> w854
                  tunnel: [1 ("index") 0 ("index")] -> w855
                  frame False {
                    n463 = property on="ValorSobrecargaC2" class="DigNum (strict)"() -> ("Value"=w864:dbl)  [unwired: 2 in, 2 out]
                    n464 = property on="UnidadesF_C2" class="Ring (strict)"() -> ("StringsAndValues[]"=w863:T6)  [unwired: 2 in, 2 out]
                  }
                  frame True {
                    n465 = property on="UnidadesF_C1" class="Ring (strict)"() -> ("StringsAndValues[]"=w865:T6)  [unwired: 2 in, 2 out]
                    n466 = property on="ValorSobrecargaC1" class="DigNum (strict)"() -> ("Value"=w867:dbl)  [unwired: 2 in, 2 out]
                  }
                }
                n467 = property on="ConversioUnitatsF" class="Arr (strict)"() -> ("Value"=w860:dbl[])  [unwired: 2 in, 2 out]
                n468 = property on="Calibratge" class="Arr (strict)"() -> ("Value"=w861:dbl[])  [unwired: 2 in, 2 out]
                n469 = Index Array(array=w861, index=w855) -> (element=w859:dbl)
                n470 = Multiply(x=w860, y=w859) -> (x*y=w858:dbl[])
                n471 = property class="Arr (strict)"(reference=w857, "Value"=w858) -> ()  [unwired: 1 in, 2 out]
                n472 = Index Array(array=w853, index=0) -> (element=w851:cluster{"String":string, "Value":u16})
                n473 = property on="Valor de control sobrecarga" class="DigNum (strict)"("Value"=w854) -> ()  [unwired: 2 in, 2 out]
                n474 = Unbundle By Name(w851) -> ("Value"=w850:u16)
                n475 = property on="UnidadesF" class="Ring (strict)"("StringsAndValues[]"=w853, "Val(Sgnl)"=w850) -> ()  [unwired: 2 in, 2 out]
              }
            }
          }
          event "CaptadorD": Value Change {
            n476 = event-data() -> ("NewVal"=w869:u16)  [unwired: 1 in, 5 out]
            n477 = property on="Calibratge D" class="Arr (strict)"() -> ("Value"=w877:dbl[])  [unwired: 2 in, 2 out]
            n478 = property on="ConversioUnitatsD" class="Arr (strict)"() -> ("Value"=w878:dbl[])  [unwired: 2 in, 2 out]
            n479 = Index Array(array=w877, index=w869) -> (element=w882:dbl)
            n480 = Multiply(x=w878, y=w882) -> (x*y=w881:dbl[])
            n481 = property on="CaptadorD" class="Ring (strict)"() -> ("StringsAndValues[]"=w876:T6)  [unwired: 2 in, 2 out]
            n482 = property on="UnidadesD" class="Ring (strict)"("Value"=w869) -> ("StringsAndValues[]"=w874:T6)  [unwired: 2 in, 2 out]
            n483 = property class="Arr (strict)"(reference=w879, "Value"=w881) -> ()  [unwired: 1 in, 2 out]
            n484 = Index Array(array=w876, index=w869) -> (element=w875:cluster{"String":string, "Value":u16})
            n485 = Index Array(array=w874, index=w869) -> (element=w873:cluster{"String":string, "Value":u16})
            n486 = Unbundle By Name(w875) -> ("String"=w868:string)
            n487 = Unbundle By Name(w873) -> ("String"=w870:string)
            n488 = Concatenate Strings(w868, " - " ("string"), w870) -> (w872:string)
            n489 = property on="Deformacion" class="DigNum (strict)"("Caption.Text"=w868) -> ()  [unwired: 2 in, 2 out]
            n490 = property class="XYGraph (strict)"("XScale.NameLbl.Text"=w872) -> ()  [unwired: 2 in, 2 out]
          }
          event "Paro Emergencia": Value Change {
            n491 = event-data() -> ("NewVal"=w887:bool)  [unwired: 1 in, 5 out]
            n492 = property on="StringsEstatMáquina" class="Arr (strict)"() -> ("Value"=w884:string[])  [unwired: 2 in, 2 out]
            n493 = property on="CodiAturada" class="DigNum (strict)"() -> ("Value"=w883:u32)  [unwired: 2 in, 2 out]
            n494 = case shown="True" w887 {
              tunnel: [w889 w893] -> w885
              tunnel: w886 -> [_ w898]
              tunnel: w884 -> [w890 w892]
              tunnel: w883 -> [w888 w891]
              frame False {
                n495 = Index Array(array=w890, index=w888) -> (element=w889:string)
              }
              frame True {
                n496 = property on="ParoProcessat" class="Bool (strict)"(reference=w898, "Value"=TRUE) -> ()  [unwired: 1 in, 2 out]
                n497 = property on="Procesa datos" class="Bool (strict)"("Value"=FALSE ("Procesa datos")) -> (error out=w896:errorcluster)  [unwired: 2 in, 1 out]
                n498 = property on="Iniciar / Finalizar" class="Bool (strict)"() -> ("Value"=w894:bool)  [unwired: 2 in, 2 out]
                n499 = Index Array(array=w892, index=w891) -> (element=w893:string)
                n500 = case shown="True" w894 {
                  tunnel: w896 -> [_ w900]
                  frame False {
                  }
                  frame True {
                    n501 = property on="Iniciar / Finalizar" class="Bool (strict)"(error in=w900, "Val(Sgnl)"=FALSE ("Value (Signaling)")) -> ()  [unwired: 1 in, 2 out]
                  }
                }
              }
            }
            n502 = property on="Estado ensayo:" class="Str"("Value"=w885) -> ()  [unwired: 2 in, 2 out]
          }
          event "BtTaraD": Value Change {
            n503 = event-data() -> ()  [unwired: 1 in, 6 out]
            n504 = property class="DigNum (strict)"(reference=w904) -> (error out=w903:errorcluster, "Value"=w902:sgl)  [unwired: 1 in, 1 out]
            n505 = property class="DigNum (strict)"(reference=w901, error in=w903, "Value"=w902) -> ()  [unwired: 2 out]
          }
          event "BtTaraF": Value Change {
            n506 = event-data() -> ()  [unwired: 1 in, 6 out]
            n507 = property class="DigNum (strict)"(reference=w907) -> ("Value"=w905:sgl)  [unwired: 1 in, 2 out]
            n508 = property class="DigNum (strict)"(reference=w906, "Value"=w905) -> ()  [unwired: 1 in, 2 out]
          }
        }
        n509 = property on="Stop" class="Bool (strict)"() -> ("Value"=w722:bool)  [unwired: 2 in, 2 out]
      }
      n510 = call <vilib>:"DAQmx Stop Task.vi"("task/channels in"=w242, "error in"=w243) -> ("task out"=w245:refnum<k21>, "error out"=w244:errorcluster)  [unwired: 12 in]
      n511 = call <vilib>:"DAQmx Stop Task.vi"("task/channels in"=w250, "error in"=w249) -> ("task out"=w252:refnum<k21>, "error out"=w251:errorcluster)  [unwired: 12 in]
      n512 = call <vilib>:"DAQmx Clear Task.vi"("task in"=w245, "error in"=w244) -> ()  [unwired: 13 in, 1 out]
      n513 = control-ref of="Pujar"() -> (w226:refnum<vi>)
      n514 = call <vilib>:"DAQmx Clear Task.vi"("task in"=w252, "error in"=w251) -> ()  [unwired: 13 in, 1 out]
      n515 = control-ref of="Salir"() -> (w256:refnum<vi>)
      n516 = control-ref of="VelocitatMàxima"() -> (w228:refnum<vi>)
      n517 = control-ref of="Velocidad Retorno"() -> (w215:refnum<vi>)
      n518 = control-ref of="Velocidad Ensayo"() -> (w216:refnum<vi>)
      n519 = control-ref of="Active_motor"() -> (w227:refnum<vi>)
      n520 = control-ref of="Ensayo activo"() -> (w206:refnum<vi>)
      n521 = control-ref of="Baixar"() -> (w225:refnum<vi>)
      n522 = control-ref of="MotorBipolar"() -> (w224:refnum<vi>)
      n523 = call "SortidaAnalogicaUSB.vi"("VelocitatAssaig"=w216, "MotorActiu"=w227, "MotorBipolar"=w224, "stop"=w256, "Pujar"=w226, "Baixar"=w225, "VelocitatRetorn"=w215, "VelocitatMaxima"=w228, "AssaigActiu"=w206) -> ()  [unwired: 7 in]
      n524 = case shown="True" TRUE {
        frame False {
        }
        frame True {
          w288 = StateEsclatometre."Initialize"  # Initial State
          # "The state machine will stop if an error occurs. If you want to handle errors in a more sophisticated way, consider adding an \"Error\" state that will process errors that occur during other states."
          n525 = control-ref of="FCI"() -> (w291:refnum<vi>)
          n526 = control-ref of="Paro Manual"() -> (w290:refnum<vi>)
          n527 = control-ref of="Cilindre"() -> (w285:refnum<vi>)
          n528 = control-ref of="LedAssaig"() -> (w286:refnum<vi>)
          n529 = control-ref of="Calibrar"() -> (w284:refnum<vi>)
          n530 = control-ref of="Baixar"() -> (w287:refnum<vi>)
          n531 = control-ref of="Pujar"() -> (w289:refnum<vi>)
          n532 = while {
            shift-right: [w308] -> _
            shift-left: T1 {"Boolean <Replace Me>"=FALSE, "String <Replace Me>"="", "Numeric <Replace Me>"=0.0} ("Data") -> [w309]
            shift-right: [w305] -> _
            shift-left: errorcluster {"status"=FALSE, "code"=0, "source"=""} ("error constant") -> [w307]
            tunnel: w291 -> [w304]
            tunnel: w290 -> [w303]
            tunnel: w289 -> [w302]
            shift-right: [w300] -> _
            shift-left: w288 -> [w301]
            tunnel: w287 -> [w299]
            tunnel: w286 -> [w298]
            tunnel: w285 -> [w296]
            tunnel: w284 -> [w295]
            stop <- w306 stop-if-true
            # "Main VI State Machine"
            n533 = property class="Bool (strict)"(reference=w295) -> ("Value"=w294:bool)  [unwired: 1 in, 2 out]
            n534 = case shown="False" w294 {
              tunnel: w309 -> [w322 w504]
              tunnel: [w321 w504] -> w308
              tunnel: w307 -> [w320 w506]
              tunnel: [w319 w506] -> w305
              tunnel: w304 -> [w318 _]
              tunnel: w303 -> [w317 _]
              tunnel: w302 -> [w316 _]
              tunnel: w301 -> [w315 _]
              tunnel: [w314 StateEsclatometre."Initialize" ("(Value Not Used)")] -> w300
              tunnel: w299 -> [w313 _]
              tunnel: w298 -> [w312 _]
              tunnel: [w311 w505] -> w297
              tunnel: w296 -> [w310 _]
              frame False {
                n535 = case shown="\"Wait for Event\"" w315 {
                  tunnel: w322 -> [w324 w356 w397 w409 w435 w455 w491 w503]
                  tunnel: [w323 w355 w395 w408 w434 w455 w491 w503] -> w321
                  tunnel: w320 -> [w332 w354 w399 w411 w438 w454 w490 w502]
                  tunnel: [w332 w353 w399 w411 w438 w454 w490 w502] -> w319
                  tunnel: w318 -> [w331 w349 _ w403 _ w451 _ _]
                  tunnel: w317 -> [w330 w348 _ _ _ w450 _ _]
                  tunnel: w316 -> [_ w351 _ w407 _ w453 w489 w500]
                  tunnel: [w328 w352 StateEsclatometre."Wait for Event" ("(Value Not Used)") w410 StateEsclatometre."Wait for Event" ("(Value Not Used)") StateEsclatometre."EsperaAssaig" ("(Value Not Used)") StateEsclatometre."Wait for Event" ("(Value Not Used)") w501] -> w314
                  tunnel: w313 -> [w327 w350 _ w401 _ w452 w488 w499]
                  tunnel: w312 -> [_ _ w394 w406 _ _ w485 w496]
                  tunnel: [w326 w347 FALSE ("Stop Loop?") FALSE ("Stop Loop?") FALSE ("Stop Loop?") FALSE ("Stop Loop?") FALSE ("Stop Loop?") w495] -> w311
                  tunnel: w310 -> [_ _ _ w404 _ w441 w482 w494]
                  frame "Initialize" {
                    w328 = StateEsclatometre."EsperaAssaig"  # Next State
                    w326 = FALSE  # Stop Loop?
                    # "Initialize - Initialize the application."
                    n536 = flat-sequence {
                      tunnel: w331 -> [w336]
                      tunnel: w330 -> [w335]
                      tunnel: w327 -> [w334]
                      tunnel: [w333] -> w329
                      tunnel: w329 -> [w346]
                      frame #0 {
                        n537 = while {
                          tunnel: w336 -> [w344]
                          tunnel: w335 -> [w343]
                          tunnel: w334 -> [w340]
                          tunnel: [w338] -> w333
                          stop <- w341 stop-if-true
                          n538 = property class="Bool (strict)"(reference=w344) -> ("Value"=w337:bool)  [unwired: 1 in, 2 out]
                          n539 = property class="Bool (strict)"(reference=w343) -> ("Value"=w342:bool)  [unwired: 1 in, 2 out]
                          n540 = property class="Bool (strict)"(reference=w340, "Value"=TRUE) -> (reference out=w338:refnum<vi>)  [unwired: 1 in, 1 out]
                          n541 = Or(x=w337, y=w342) -> (x .or. y?=w341:bool)
                        }
                      }
                      frame #1 {
                        n542 = property class="Bool (strict)"(reference=w346, "Value"=FALSE) -> ()  [unwired: 1 in, 2 out]
                      }
                    }
                    n543 = Bundle By Name(cluster=w324, "String <Replace Me>"="Anar a Pos Ini") -> (w323:T1)
                  }
                  frame "Wait for Event" {
                    # "Wait for Event - Use an Event Structure to monitor the user interface for events that run different states of the state machine."
                    n544 = event shown="[5] \"IniciAssaig\": Value Change" {
                      selector: _ -> [_ _ _ _ _ _]
                      dyn-events: _ -> [_ _ _ _ _ _]
                      timeout: _ -> [_ _ _ _ _ _]
                      tunnel: [w361 StateEsclatometre."Exit" ("Initial State") w371 w373 w380 w387] -> w352
                      tunnel: w356 -> [w358 w363 w368 w376 w378 w391]
                      tunnel: [w357 w362 w367 w376 w377 w390] -> w355
                      tunnel: w354 -> [w360 w366 w372 w375 w383 w388]
                      tunnel: [w360 w366 w372 w375 w383 w388] -> w353
                      tunnel: w351 -> [_ _ _ _ _ _]
                      tunnel: w350 -> [_ _ _ _ _ _]
                      tunnel: w349 -> [_ _ _ _ _ _]
                      tunnel: w348 -> [_ _ _ _ _ _]
                      tunnel: [_ _ _ _ w382 _] -> w347
                      event "Stop": Value Change {
                        w361 = StateEsclatometre."Exit"  # Next State
                        n545 = event-data() -> ()  [unwired: 1 in, 1 out]
                        n546 = Bundle By Name(cluster=w358, "String <Replace Me>"="STOP" ("Running User State 1")) -> (w357:T1)
                      }
                      event "Salir": Value Change {
                        n547 = event-data() -> ()  [unwired: 1 in, 1 out]
                        n548 = Bundle By Name(cluster=w363, "String <Replace Me>"="SALIR" ("Running User State 1")) -> (w362:T1)
                      }
                      event "Paro Manual", "FCS", "Sobrecarga": Value Change {
                        w371 = StateEsclatometre."FiAssaig"  # Initial State
                        n549 = event-data() -> ()  [unwired: 1 in, 4 out]
                        n550 = property on="Iniciar / Finalizar" class="Bool (strict)"("Val(Sgnl)"=FALSE ("Value (Signaling)")) -> ()  [unwired: 2 in, 2 out]
                        n551 = Bundle By Name(cluster=w368, "String <Replace Me>"="PARO_MAN-FCS-SOBRE" ("Running User State 1")) -> (w367:T1)
                      }
                      event "Paro Emergencia": Value Change {
                        w373 = StateEsclatometre."Emergencia"  # Initial State
                        n552 = event-data() -> ()  [unwired: 1 in, 6 out]
                        n553 = property on="Iniciar / Finalizar" class="Bool (strict)"("Val(Sgnl)"=FALSE ("Value (Signaling)")) -> ()  [unwired: 2 in, 2 out]
                      }
                      event "ParoRotura": Value Change {
                        w382 = FALSE  # Stop Loop?
                        w380 = StateEsclatometre."FiAssaig"  # Initial State
                        n554 = event-data() -> ("NewVal"=w381:bool)  [unwired: 1 in, 4 out]
                        n555 = case shown="True" w381 {
                          frame False {
                          }
                          frame True {
                            n556 = property on="Procesa datos" class="Bool (strict)"("Value"=FALSE ("Procesa datos")) -> (error out=w386:errorcluster)  [unwired: 2 in, 1 out]
                            n557 = property on="Iniciar / Finalizar" class="Bool (strict)"(error in=w386, "Val(Sgnl)"=FALSE ("Value (Signaling)")) -> ()  [unwired: 1 in, 2 out]
                          }
                        }
                        n558 = Bundle By Name(cluster=w378, "String <Replace Me>"="ROTURA" ("Running User State 1")) -> (w377:T1)
                      }
                      event "IniciAssaig": Value Change {
                        w387 = StateEsclatometre."IniciaAssaig"  # Initial State
                        n559 = event-data() -> ()  [unwired: 1 in, 1 out]
                        n560 = Bundle By Name(cluster=w391, "String <Replace Me>"="PremBotoInici" ("Running User State 1")) -> (w390:T1)
                      }
                    }
                  }
                  frame "EsperaAssaig", Default {
                    n561 = property class="Bool (strict)"(reference=w394, "Value"=TRUE) -> ()  [unwired: 1 in, 2 out]
                    n562 = Bundle By Name(cluster=w397, "String <Replace Me>"="EsperaAssaig") -> (w395:T1)
                  }
                  frame "IniciaAssaig" {
                    # "User State 2 - Replace this state with functionality for your own application."
                    n563 = property class="Bool (strict)"(reference=w403) -> ("Value"=w402:bool)  [unwired: 1 in, 2 out]
                    n564 = case shown="True" w402 {
                      tunnel: [w414 w422] -> w410
                      tunnel: w407 -> [_ w421]
                      tunnel: w406 -> [_ w420]
                      tunnel: w404 -> [_ w419]
                      tunnel: w401 -> [_ w418]
                      tunnel: ["Incialitzarà" ("String <Replace Me>") "IniciaAssaig" ("String <Replace Me>")] -> w400
                      frame False {
                        n565 = property on="Ensayo activo" class="Bool (strict)"() -> ("Value"=w412:bool)  [unwired: 2 in, 2 out]
                        n566 = case shown="True" w412 {
                          tunnel: [w415 w416] -> w414
                          frame False {
                            w415 = StateEsclatometre."Initialize"  # Next State
                          }
                          frame True {
                            w416 = StateEsclatometre."Wait for Event"  # Next State
                          }
                        }
                      }
                      frame True {
                        w422 = StateEsclatometre."Assaig"  # Next State
                        n567 = flat-sequence {
                          tunnel: w420 -> [w425]
                          tunnel: w419 -> [w423]
                          tunnel: w421 -> [w431]
                          tunnel: w418 -> [w430]
                          frame #0 {
                            n568 = property class="Bool (strict)"(reference=w425, "Value"=FALSE) -> ()  [unwired: 1 in, 2 out]
                            n569 = property class="Bool (strict)"(reference=w423, "Value"=TRUE) -> ()  [unwired: 1 in, 2 out]
                          }
                          frame #1 {
                            n570 = Wait Until Next ms Multiple(millisecond multiple=u32 1000) -> ()  [unwired: 1 out]
                          }
                          frame #2 {
                            n571 = property class="Bool (strict)"(reference=w430, "Value"=FALSE) -> ()  [unwired: 1 in, 2 out]
                            n572 = property on="Iniciar / Finalizar" class="Bool (strict)"("Val(Sgnl)"=TRUE ("Value (Signaling)")) -> ()  [unwired: 2 in, 2 out]
                            n573 = property class="Bool (strict)"(reference=w431, "Value"=TRUE) -> ()  [unwired: 1 in, 2 out]
                          }
                        }
                      }
                    }
                    n574 = Bundle By Name(cluster=w409, "String <Replace Me>"=w400) -> (w408:T1)
                  }
                  frame "Assaig" {
                    n575 = Bundle By Name(cluster=w435, "String <Replace Me>"="Assaig") -> (w434:T1)
                  }
                  frame "FiAssaig" {
                    n576 = flat-sequence {
                      tunnel: w452 -> [w461]
                      tunnel: [w459] -> w444
                      tunnel: w451 -> [w458]
                      tunnel: [w458] -> w443
                      tunnel: w450 -> [_]
                      tunnel: w453 -> [w457]
                      tunnel: [w456] -> w442
                      tunnel: w441 -> [w456]
                      tunnel: w444 -> [w465]
                      tunnel: [w465] -> w446
                      tunnel: w443 -> [w464]
                      tunnel: [w464] -> w445
                      tunnel: w442 -> [w462]
                      tunnel: [w462] -> w439
                      tunnel: w446 -> [w469]
                      tunnel: w445 -> [w468]
                      tunnel: [w467] -> w449
                      tunnel: [w466] -> w440
                      tunnel: w439 -> [w466]
                      tunnel: w449 -> [w478]
                      tunnel: w440 -> [w475]
                      frame #0 {
                        w460 = FALSE ("Value")
                        n577 = property class="Bool (strict)"(reference=w457, "Value"=w460) -> ()  [unwired: 1 in, 2 out]
                        n578 = property class="Bool (strict)"(reference=w461, "Value"=w460) -> (reference out=w459:refnum<vi>)  [unwired: 1 in, 1 out]
                      }
                      frame #1 {
                        n579 = Wait Until Next ms Multiple(millisecond multiple=u32 500) -> ()  [unwired: 1 out]
                      }
                      frame #2 {
                        n580 = while {
                          tunnel: w468 -> [w474]
                          tunnel: w469 -> [w473]
                          tunnel: [w471] -> w467
                          stop <- w470 stop-if-true
                          n581 = property class="Bool (strict)"(reference=w474) -> ("Value"=w470:bool)  [unwired: 1 in, 2 out]
                          n582 = property class="Bool (strict)"(reference=w473, "Value"=TRUE) -> (reference out=w471:refnum<vi>)  [unwired: 1 in, 1 out]
                        }
                      }
                      frame #3 {
                        n583 = property class="Bool (strict)"(reference=w478, "Value"=FALSE) -> ()  [unwired: 1 in, 2 out]
                        n584 = property class="Bool (strict)"(reference=w475, "Value"=FALSE) -> ()  [unwired: 1 in, 2 out]
                      }
                      frame #4 {
                        n585 = Wait Until Next ms Multiple(millisecond multiple=u32 500) -> ()  [unwired: 1 out]
                      }
                    }
                  }
                  frame "Emergencia" {
                    w484 = FALSE ("Value")
                    n586 = property class="Bool (strict)"(reference=w489, "Value"=w484) -> ()  [unwired: 1 in, 2 out]
                    n587 = property class="Bool (strict)"(reference=w488, "Value"=w484) -> ()  [unwired: 1 in, 2 out]
                    n588 = property class="Bool (strict)"(reference=w485, "Value"=FALSE) -> ()  [unwired: 1 in, 2 out]
                    n589 = property class="Bool (strict)"(reference=w482) -> (reference out=w480:refnum<vi>, "Value"=w481:bool)  [unwired: 1 in, 1 out]
                    n590 = case shown="False" w481 {
                      tunnel: w480 -> [w492 _]
                      frame False {
                        n591 = property class="Bool (strict)"(reference=w492, "Value"=FALSE) -> ()  [unwired: 1 in, 2 out]
                      }
                      frame True {
                      }
                    }
                  }
                  frame "Exit" {
                    w497 = FALSE ("Value")
                    w498 = FALSE ("Value")
                    w495 = TRUE  # Stop Loop?
                    w501 = StateEsclatometre."Exit"  # (Value Not Used)
                    # "Exit - Exit the application."
                    n592 = property class="Bool (strict)"(reference=w500, "Value"=w498) -> ()  [unwired: 1 in, 2 out]
                    n593 = property class="Bool (strict)"(reference=w499, "Value"=w498) -> ()  [unwired: 1 in, 2 out]
                    n594 = property class="Bool (strict)"(reference=w494, "Value"=w497) -> ()  [unwired: 1 in, 2 out]
                    n595 = property class="Bool (strict)"(reference=w496, "Value"=w497) -> ()  [unwired: 1 in, 2 out]
                  }
                }
              }
              frame True {
                n596 = property on="Stop" class="Bool (strict)"() -> ("Value"=w505:bool)  [unwired: 2 in, 2 out]
              }
            }
            "Data" <- w308
            n597 = Or(x=w305, y=w297) -> (x .or. y?=w306:bool)
          }
        }
      }
      n598 = Unregister For Events(event registration refnum=w232) -> ()  [unwired: 1 in, 1 out]
      n599 = Current VI's Menubar() -> (w282:refnum<k9>)
      n600 = Delete Menu Items(9:w282) -> (3:w281:refnum<k9>)  [unwired: 3 in, 1 out]
      n601 = Insert Menu Items(8:string[] ["Calibra", "About"] ("item names"), 9:w281) -> (3:w230:refnum<k9>)  [unwired: 4 in, 2 out]
      n602 = while {
        tunnel: w230 -> [w620]
        stop <- w619 stop-if-true
        n603 = Get Menu Selection(0:w620, 1:200 ("ms timeout (200)")) -> (6:w621:string)  [unwired: 2 in, 4 out]
        n604 = case shown="\"Calibra\"" w621 {
          frame "About" {
            n605 = call "About.vi"() -> ()  [unwired: 1 in]
          }
          frame "Calibra" {
            n606 = control-ref of="Password"() -> (w625:refnum<vi>)
            n607 = property class="Str"(reference=w625) -> ("Value"=w624:string)  [unwired: 1 in, 2 out]
            n608 = call "Password.vi"() -> ("Password"=w626:string)  [unwired: 17 in, 2 out]
            n609 = Equal?(x=w624, y=w626) -> (x = y?=w623:bool)
            n610 = case shown="True" w623 {
              frame False {
              }
              frame True {
                n611 = call "Calibratge.vi"() -> ("OK ?"=w627:bool)  [unwired: 10 in]
                n612 = case shown="True" w627 {
                  frame False {
                  }
                  frame True {
                    n613 = control-ref of="Valor de control sobrecarga"() -> (w641:refnum<vi>)
                    n614 = call "ReadCal.vi"() -> ("SobrecargaC2"=w639:dbl, "ResoExten"=w647:i8, "TextTemps"=w657:string, "TextDefor"=w656:string, "SegonCaptador"=w668:string, "MotorBipolar"=w635:bool, "UnitatsC2"=w677:string, "UnitatsC1"=w679:string, "PrimerCaptador"=w669:string, "ViuMotor"=w633:bool, "DeforActiva"=w637:bool, "Unidades"=w629:u8, "Calibrar"=w632:bool, "SobrecargaC1"=w640:dbl, "Password"=w692:string, "Pendents"=w652:dbl[], "VelocitatMàxima"=w645:dbl)  [unwired: 2 in, 9 out]
                    n615 = property on="ResoExten" class="Ring (strict)"("Value"=w647) -> ()  [unwired: 2 in, 2 out]
                    n616 = control-ref of="ValorSobrecargaC1"() -> (w644:refnum<vi>)
                    n617 = control-ref of="ValorSobrecargaC2"() -> (w643:refnum<vi>)
                    n618 = Decimal String To Number(string=w668) -> (number=w674:i32)  [unwired: 2 in, 1 out]
                    n619 = property class="DigNum (strict)"(reference=w643, "Value"=w639) -> ()  [unwired: 1 in, 2 out]
                    n620 = Decimal String To Number(string=w669) -> (number=w675:i32)  [unwired: 2 in, 1 out]
                    n621 = control-ref of="ViuMotor"() -> (w634:refnum<vi>)
                    n622 = property on="Células" class="Ring (strict)"() -> ("StringsAndValues[]"=w673:T5)  [unwired: 2 in, 2 out]
                    n623 = property class="DigNum (strict)"(reference=w644, "Value"=w640) -> ()  [unwired: 1 in, 2 out]
                    n624 = control-ref of="DeforActiu"() -> (w638:refnum<vi>)
                    n625 = property class="Bool (strict)"(reference=w638, "Value"=w637) -> ()  [unwired: 1 in, 2 out]
                    n626 = control-ref of="MotorBipolar"() -> (w636:refnum<vi>)
                    n627 = property class="Bool (strict)"(reference=w634, "Value"=w633) -> ()  [unwired: 1 in, 2 out]
                    n628 = property class="Bool (strict)"(reference=w636, "Value"=w635) -> ()  [unwired: 1 in, 2 out]
                    n629 = property on="CaptadorF" class="Ring (strict)"() -> ("Value"=w642:u16)  [unwired: 2 in, 2 out]
                    n630 = property on="Calibrar" class="Bool (strict)"("Value"=w632) -> ()  [unwired: 2 in, 2 out]
                    n631 = case shown="0, Default" w642 {
                      tunnel: w641 -> [w694 w696]
                      tunnel: w640 -> [w693 _]
                      tunnel: w639 -> [_ w695]
                      frame 0, Default {
                        n632 = property class="DigNum (strict)"(reference=w694, "Value"=w693) -> ()  [unwired: 1 in, 2 out]
                      }
                      frame 1 {
                        n633 = property class="DigNum (strict)"(reference=w696, "Value"=w695) -> ()  [unwired: 1 in, 2 out]
                      }
                    }
                    n634 = control-ref of="ArraiUnitats"() -> (w678:refnum<vi>)
                    n635 = Index Array(array=w673, index=w675) -> (element=w667:cluster{"String":string, "Value":u8})
                    n636 = Index Array(array=w673, index=w674) -> (element=w671:cluster{"String":string, "Value":u8})
                    n637 = control-ref of="Pendents"() -> (w690:refnum<vi>)
                    n638 = property class="Arr (strict)"(reference=w690, "Value"=w652) -> ()  [unwired: 1 in, 2 out]
                    n639 = Unbundle(w667) -> ("Value"=w666:u8)  [unwired: 1 out]
                    n640 = control-ref of="VelocitatMàxima"() -> (w646:refnum<vi>)
                    n641 = property class="DigNum (strict)"(reference=w646, "Value"=w645) -> ()  [unwired: 1 in, 2 out]
                    n642 = call "UnitatsStringsValors.vi"("UnitatsC1"=w679, "Arr Refnum"=w678) -> ("Array 2"=w630:cluster{"String":string, "Value":u16}[])  [unwired: 1 out]
                    n643 = call "UnitatsStringsValors.vi"("UnitatsC1"=w677, "Arr Refnum"=w678) -> ("Array 2"=w676:cluster{"String":string, "Value":u16}[])  [unwired: 1 out]
                    n644 = property on="Activa cilindre" class="Bool (strict)"("Value"=FALSE ("ActivaCilindre"), "Visible"=w632) -> ()  [unwired: 2 in, 2 out]
                    n645 = property on="Password" class="Str"("Value"=w692) -> ()  [unwired: 2 in, 2 out]
                    n646 = Unbundle(w671) -> ("Value"=w670:u8)  [unwired: 1 out]
                    n647 = property on="Celula_0" class="DigNum (strict)"("Value"=w666) -> ()  [unwired: 2 in, 2 out]
                    n648 = property on="UnidadesF_C2" class="Ring (strict)"("StringsAndValues[]"=w676) -> ()  [unwired: 2 in, 2 out]
                    n649 = case shown="0, Default" w670 {
                      tunnel: w667 -> [w704 w705]
                      tunnel: w671 -> [w703 _]
                      tunnel: [w702 w706] -> w672
                      frame 0, Default {
                        n650 = Build Array(w704, w703) -> (w702:cluster{"String":string, "Value":u8}[])
                      }
                      frame 17 {
                        n651 = Build Array(w705) -> (w706:cluster{"String":string, "Value":u8}[])
                      }
                    }
                    n652 = property on="DeforActiu" class="Bool (strict)"() -> ("Value"=w628:bool)  [unwired: 2 in, 2 out]
                    n653 = Index Array(array=w652, index=2) -> (element=w683:dbl)
                    n654 = Index Array(array=w652, index=0) -> (element=w684:dbl)
                    n655 = Index Array(array=w652, index=1) -> (element=w660:dbl)
                    n656 = Index Array(array=w652, index=3) -> (element=w659:dbl)
                    n657 = property on="UnidadesF_C1" class="Ring (strict)"("StringsAndValues[]"=w630) -> ()  [unwired: 2 in, 2 out]
                    n658 = control-ref of="ConversioUnitatsD"() -> (w665:refnum<vi>)
                    n659 = Build Array(w684, w683) -> (w681:dbl[])
                    n660 = control-ref of="Calibratge"() -> (w682:refnum<vi>)
                    n661 = Build Array(w660, w659) -> (w658:dbl[])
                    n662 = case shown="True" w628 {
                      tunnel: w657 -> [w697 w700]
                      tunnel: w656 -> [_ w699]
                      tunnel: [w698 w701] -> w655
                      frame False {
                        (unwired) FALSE ("Extensometre")
                        n663 = Build Array(w697) -> (w698:string[])
                      }
                      frame True {
                        n664 = Build Array(w700, w699) -> (w701:string[])
                      }
                    }
                    n665 = control-ref of="ConversioUnitatsF"() -> (w691:refnum<vi>)
                    n666 = control-ref of="Calibratge D"() -> (w663:refnum<vi>)
                    n667 = property class="Arr (strict)"(reference=w665) -> ("Value"=w653:dbl[])  [unwired: 1 in, 2 out]
                    n668 = property class="Arr (strict)"(reference=w682, "Value"=w681) -> ()  [unwired: 1 in, 2 out]
                    n669 = property class="Arr (strict)"(reference=w663, "Value"=w658) -> ()  [unwired: 1 in, 2 out]
                    n670 = property class="Arr (strict)"(reference=w691) -> ("Value"=w689:dbl[])  [unwired: 1 in, 2 out]
                    n671 = Index Array(array=w652, index=0) -> (element=w680:dbl)
                    n672 = property on="CaptadorD" class="Ring (strict)"("Strings []"=w655, "Value"=0 ("index")) -> ()  [unwired: 2 in, 2 out]
                    n673 = Index Array(array=w652, index=1) -> (element=w651:dbl)
                    n674 = property on="CaptadorF" class="Ring (strict)"("StringsAndValues[]"=w672, "Value"=w666) -> ()  [unwired: 2 in, 2 out]
                    n675 = Multiply(x=w689, y=w680) -> (x*y=w687:dbl[])
                    n676 = control-ref of="FactorsUnitatsPendents_F"() -> (w688:refnum<vi>)
                    n677 = Multiply(x=w653, y=w651) -> (x*y=w650:dbl[])
                    n678 = control-ref of="FactorsUnitatsPendents_D"() -> (w664:refnum<vi>)
                    n679 = property on="UnidadesF" class="Ring (strict)"("Value"=w629, "StringsAndValues[]"=w630) -> ()  [unwired: 2 in, 2 out]
                    n680 = property class="Arr (strict)"(reference=w688, "Value"=w687) -> ()  [unwired: 1 in, 2 out]
                    n681 = property class="Arr (strict)"(reference=w664, "Value"=w650) -> ()  [unwired: 1 in, 2 out]
                  }
                }
              }
            }
          }
          frame Default {
          }
        }
        n682 = property on="Stop" class="Bool (strict)"() -> ("Value"=w619:bool)  [unwired: 2 in, 2 out]
      }
    }
    frame #5 {
      n683 = property on="rings" class="Arr (strict)"() -> ("Value"=w1184:refnum<vi>[])  [unwired: 2 in, 2 out]
      n684 = call "GuardaValorsPantalla.vi"("Rings"=w1184) -> ()  [unwired: 9 in, 1 out]
    }
    frame #6 {
      n685 = Quit LabVIEW(quit? (T)=TRUE) -> ()
    }
  }
